vi "AO_master_CorrLoop_PD_2D_v4.vi"() -> ()   [LabVIEW 2018]
uses:
  <userlib>/WaveKit.lib/Controls/Wavefront Corrector states - ONE.ctl
  <userlib>/WaveKit.lib/Classes/WavefrontCorrector/WavefrontCorrector.lvclass
  <userlib>/WaveKit.lib/Classes/WavefrontCorrectorSet/WavefrontCorrectorSet.lvclass
  <vilib>/Analysis/1siggen.llb/Ramp Pattern by Samples.vi
  <vilib>/Utility/file.llb/Read From Spreadsheet File (DBL).vi
  <vilib>/Analysis/1siggen.llb/Ramp Pattern by Delta.vi
  <vilib>/Analysis/NI_AALBase.lvlib
panel:
  in  "Status":enum32{"Page 1", "Page 2"}(tab)
  out "DM Initial State":T1[](array[typedef])
  out "Return from CheckTimings":u32
  out "Calculated Exposure Value":sgl format="%.2f"
  out "Return from SetTemperature":u32
  out "Return from Initialize":u32
  out "Detector X Pixels":i32
  out "Detector Y Pixels":i32
  in  "Tab Control":T2(tab)
  in  "Flip mirror port":tag="Dev1/ao5"
  in  "interaction matrix file":path=path "D:/SystemAlignment/IM_20220706_1p5sx2_0p5um.aomi"
  in  "Haso configuration file":path=path "C:/Program Files (x86)/Imagine Optic/Configuration Files/HASO3_first_7364.dat"
  in  "Offset command file":path=path "D:/SystemAlignment/system_aberration_20220720.dat"
  in  "Initial haso file":path=path "D:/SystemAlignment/system_aberration_residual_20220406.has"
  out "# of Phase":i32
  in  "DM configuration file":path=path "C:/Program Files (x86)/Imagine Optic/Configuration Files/WaveFrontCorrector_mirao52-e_0326.dat"
  out "DM ActuatorsNumber":i32
  out "Error out":errorcluster
  in  "EMCCD trigger port":tag="Dev1/port0/line0"
  in  "488 shutter":refnum<k7>(container)
  in  "?":bool
  out "Flip Mirror Status":sgl(ring) items=["EMCCD Camera"=-5, "Wavefront sensor"=1]
  in  "Defocus":bool=TRUE
  in  "Tilts":bool=TRUE
  in  "Max zern num":u32=14
  in  "Density":sgl=0.3 min=0 max=1 format="%#.4f"
  in  "Amplitude":sgl=0.3 min=0 format="%#.4f"
  in  "idxType":enum16{"Wyant", "ANSI"}(ring)=enum."ANSI"
  in  "Zern coeffs file":path=path "D:/SystemAlignment/system_aberration_residual_20200711.txt"
  in  "Diversity Zern Coeffs":enum16{"Manual ", "ZernFile"}(ring)
  out "Zern coeffs (random)":sgl[](array[numeric])
  out "Zern index (random)":i32[](array[numeric])
  in  "Initial Zern Coeffs":enum16{"Manual ", "Random"}(ring)
  in  "Exp Repeat Num":i32=1
  in  "Index 5":i32[](array[numeric])=[3, 4, 5, 6, 7, 8]
  in  "Coeffs 4":sgl[](array[numeric])=[0.5, -0.2, 0.0, 0.0, 0.0, 0.0]
  in  "Index 4":i32[](array[numeric])=[3, 4, 5, 6, 7, 8]
  in  "Coeffs 3":sgl[](array[numeric])=[0.0, -0.2, 0.5, 0.0, 0.0, 0.0]
  in  "Index 3":i32[](array[numeric])=[3, 4, 5, 6, 7, 8]
  in  "Coeffs 2":sgl[](array[numeric])=[0.5, 0.2, 0.0, 0.0, 0.0, 0.0]
  in  "Index 2":i32[](array[numeric])=[3, 4, 5, 6, 7, 8]
  in  "Coeffs 5":sgl[](array[numeric])=[0.0, 0.2, 0.5, 0.0, 0.0, 0.0]
  in  "Zern index initial":i32[](array[numeric])=[3, 5, 6, 7, 12]
  in  "Zern coeffs initial":sgl[](array[numeric])=[0.0, 0.4, 0.0, 0.3, 0.0]
  out "Img Num Used":dbl[](array[numeric])
  out "Corrected IQM":dbl
  out "Recon Img Num":u32=2
  out "Current Exp Num":u32=2
  in  "Auto Stop":bool=TRUE
  in  "Feedback Type":T3(ring)=enum."One Step Feedback"
  in  "Initial Phase Num":u32=2
  out "RMSE Value":dbl
  out "Recon Time (s)":dbl
  in  "File Base Name":string="beads"
  in  "Images/phase":i32=1
  in  "Exposure time (s)":dbl=0.02
  in  "Div Phase Num":i32=5
  in  "Metrics Type":T4(ring)=enum."norm DCT  - spectral domain 3: 0~r0"
  in  "Apply Defocus":bool
  in  "PD Correction":bool=TRUE
  in  "Num for average":u32=1
  in  "Zernike Index Limit":u32=20
  in  "Max Iteration Num":u32=10
  in  "Gamma Value":dbl=1e-10
  in  "Crop Size of image":u32=512
  in  "Background Value":dbl=300.0
  in  "Show Input":bool
  in  "Show Recon":bool=TRUE
  in  "Use GPU":bool=TRUE
  out "Cooling":i32
  in  "Trigger":u32(ring)=1 items=["Internal", "External"]
  in  "Cooler set to Temperature":i32=-60
  in  "Initialize EMCCD?":bool=TRUE
  in  "Turn off EMCCD when finished?":bool
  in  "Main Path":path=path "D:/Data"
  in  "Subfolder":string="Test1"
  in  "Folder Name":string="Test"
  out "Groundtruth IQM":dbl
  out "Aberrated IQM":dbl
  out "All IQM":dbl[](array[numeric])
  in  "Final Phase Num":u32=3
  out "Output path":path=path "D:/Data"
  out "Log File Path":path
  out "Zern coeffs recon":sgl[](array[numeric])
  # "AO correction loop based on phase diversity: 2D image case (last update: 20200821)\nVersion 3: A combination of LabVIEW, MATLAB (EMCCD controlled by LabVIEW) for sensorless AO with IQM feedback , modified from Version 3. New updates:\n1) fix last 2 bugs, re-organize user interface, reform program design (framework reshaped)\n2) more control to laser and EMCCD (ROI, gain, preview)"
  # "How to use\n1) Set Flip mirror to EMCCD (AO_mini_stage and shutter control.vi);\n2) Run this VI;\n3) When cooling gets to -55, the system start to acquire data."
  # "Bugs: \n1) when run this vi first time, there is big shift between diversity images. If repeat, then shift disappears.\n2) diversity image number is not controllable, always output 5 images."
  # "Andor Status"
  # "Manual input"
  # "Random input"
  # "Manual input sequence"
  # "File input"
  # "Path and File Name"
  # "Andor EMCCD Settings"
  # "AO Correction Settings"
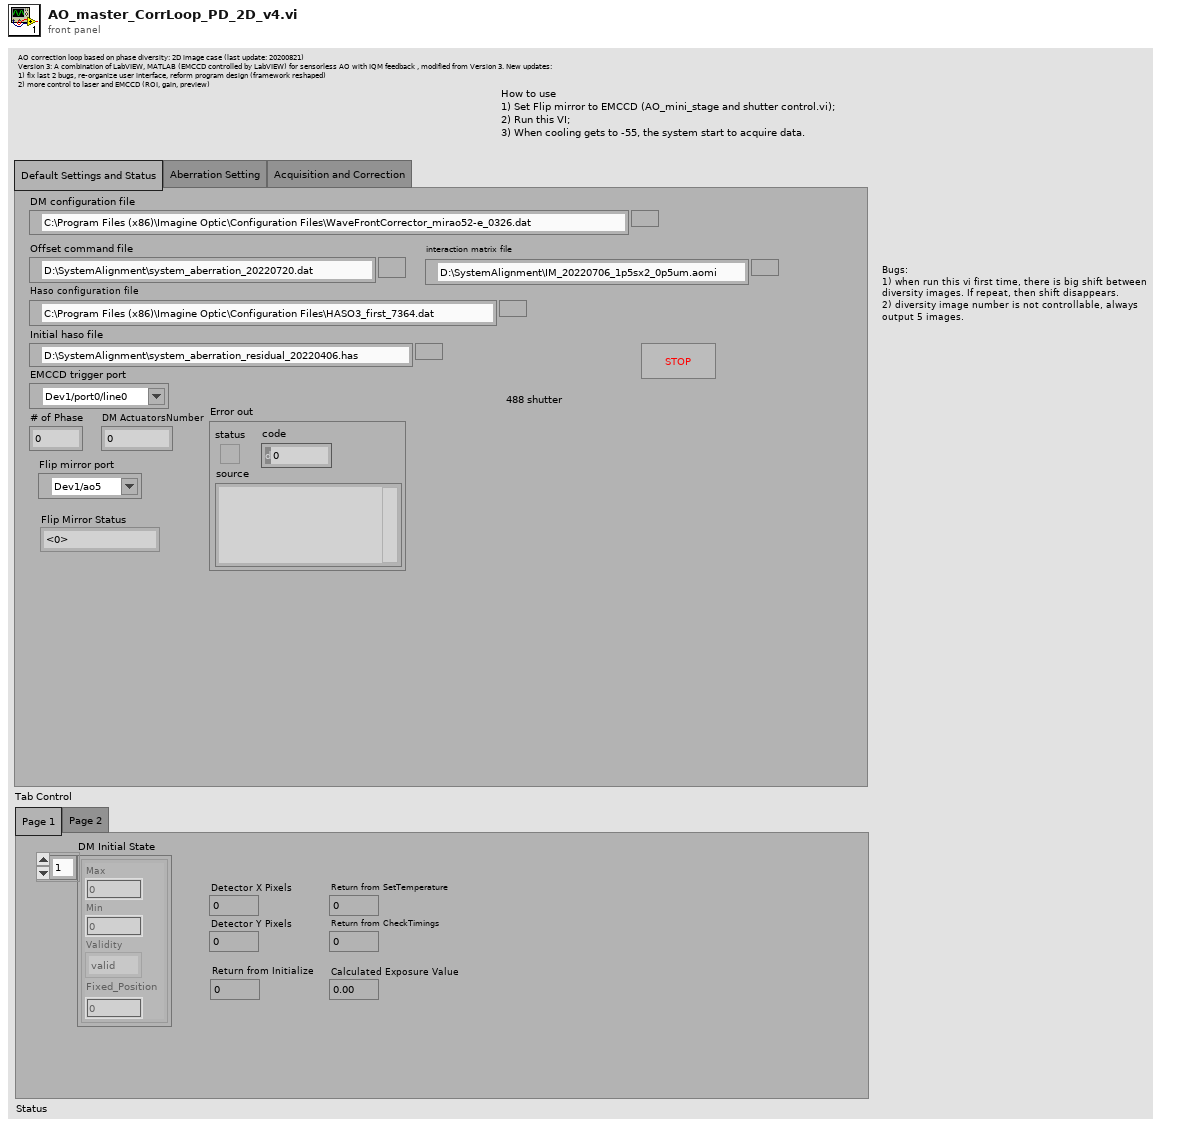
[diagram p1: front panel]
types:
  T1 = typedef "Wavefront Corrector states - ONE.ctl" = cluster{"Max":sgl, "Min":sgl, "Validity":enum16{"valid", "fixed", "invalid"}, "Fixed_Position":sgl}
  T2 = enum32{"Default Settings and Status", "Aberration Setting", "Acquisition and Correction"}
  T3 = enum16{"Single Correction", "One Step Feedback", "Progressive Feedback"}
  T4 = enum16{" ", "max intensity", "mean intensity", "RMS contrast", "sharpness - image domain", "sharpness - spectral domain 1: 0~r0", "sharpness - spectral domain 2: 0.1*r0~0.5*r0", "norm DCT  - spectral domain 3: 0~r0"}
  T5 = typedef "Error Code Enum typedef.ctl" = enum32{"N/A (0)", "DRV_ERROR_CODES", "DRV_SUCCESS", "DRV_VXDNOTINSTALLED", "DRV_ERROR_SCAN", "DRV_ERROR_CHECK_SUM", "DRV_ERROR_FILELOAD", "DRV_UNKNOWN_FUNC", "DRV_ERROR_VXD_INIT", "DRV_ERROR_ADDRESS", "DRV_ERROR_PAGELOCK", "DRV_ERROR_PAGEUNLOCK", "DRV_ERROR_BOARDTEST", "DRV_ERROR_ACK", "DRV_ERROR_UP_FIFO", "DRV_ERROR_PATTERN", "N/A (16)", "DRV_ACQUISITION_ERRORS", "DRV_ACQ_BUFFER", "DRV_ACQ_DOWNFIFO_FULL", "DRV_PROC_UNKONWN_INSTRUCTION", "DRV_ILLEGAL_OP_CODE", "DRV_KINETIC_TIME_NOT_MET", "DRV_ACCUM_TIME_NOT_MET", "DRV_NO_NEW_DATA", "N/A (25)", "DRV_SPOOLERROR", "N/A (27)", "N/A (28)", "N/A (29)", "N/A (30)", "N/A (31)", "N/A (32)", "DRV_TEMPERATURE_CODES", "DRV_TEMPERATURE_OFF", "DRV_TEMPERATURE_NOT_STABILIZED", "DRV_TEMPERATURE_STABILIZED", "DRV_TEMPERATURE_NOT_REACHED", "DRV_TEMPERATURE_OUT_RANGE", "DRV_TEMPERATURE_NOT_SUPPORTED", "DRV_TEMPERATURE_DRIFT", "N/A (41)", "N/A (42)", "N/A (43)", "N/A (44)", "N/A (45)", "N/A (46)", "N/A (47)", "N/A (48)", "DRV_GENERAL_ERRORS", "DRV_INVALID_AUX", "DRV_COF_NOTLOADED", "DRV_FPGAPROG", "DRV_FLEXERROR", "DRV_GPIBERROR", "N/A (55)", "N/A (56)", "N/A (57)", "N/A (58)", "N/A (59)", "N/A (60)", "N/A (61)", "N/A (62)", "N/A (63)", "DRV_DATATYPE", "DRV_DRIVER_ERRORS", "DRV_P1INVALID", "DRV_P2INVALID", "DRV_P3INVALID", "DRV_P4INVALID", "DRV_INIERROR", "DRV_COFERROR", "DRV_ACQUIRING", "DRV_IDLE", "DRV_TEMPCYCLE", "DRV_NOT_INITIALIZED", "DRV_P5INVALID", "DRV_P6INVALID", "DRV_INVALID_MODE", "DRV_INVALID_FILTER", "DRV_I2CERRORS", "DRV_I2CDEVNOTFOUND", "DRV_I2CTIMEOUT", "DRV_P7INVALID", "N/A (84)", "N/A (85)", "N/A (86)", "N/A (87)", "N/A (88)", "N/A (89)", "DRV_IOCERROR", "DRV_VRMVERSIONERROR"}
  T6 = typedef "NI_Matrix.lvlib/RealMatrix.ctl" = dbl[][]
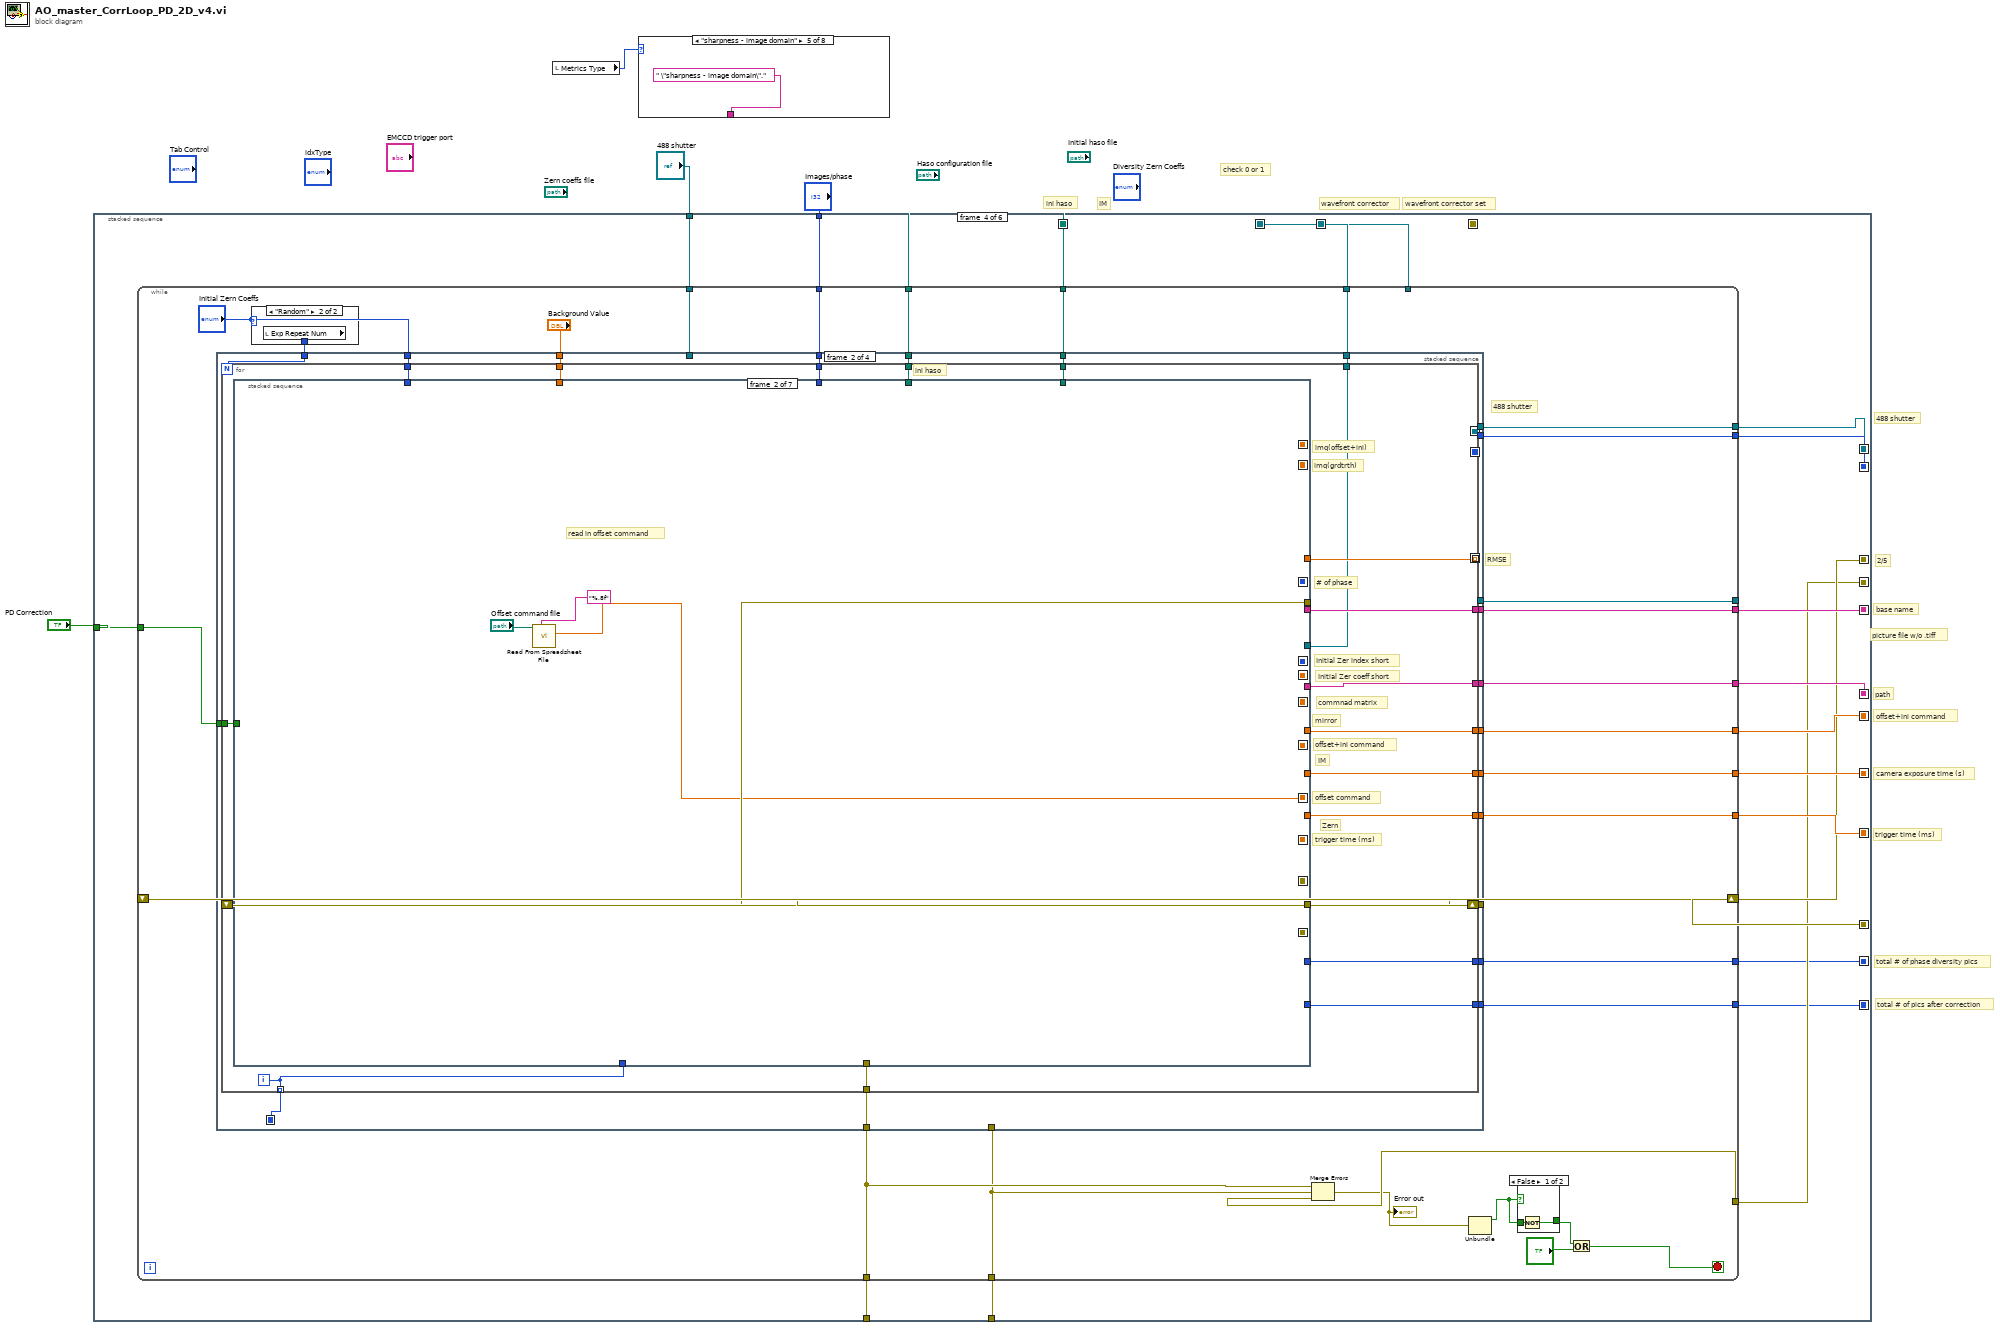
[diagram p0: block diagram]
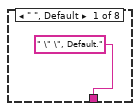
[diagram p2: hidden frame]
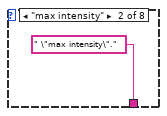
[diagram p3: hidden frame]
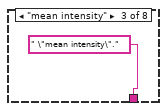
[diagram p4: hidden frame]
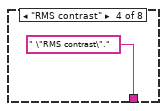
[diagram p5: hidden frame]
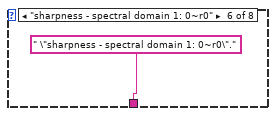
[diagram p6: hidden frame]
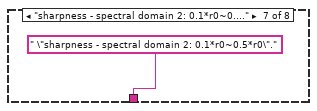
[diagram p7: hidden frame]
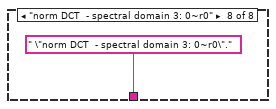
[diagram p8: hidden frame]
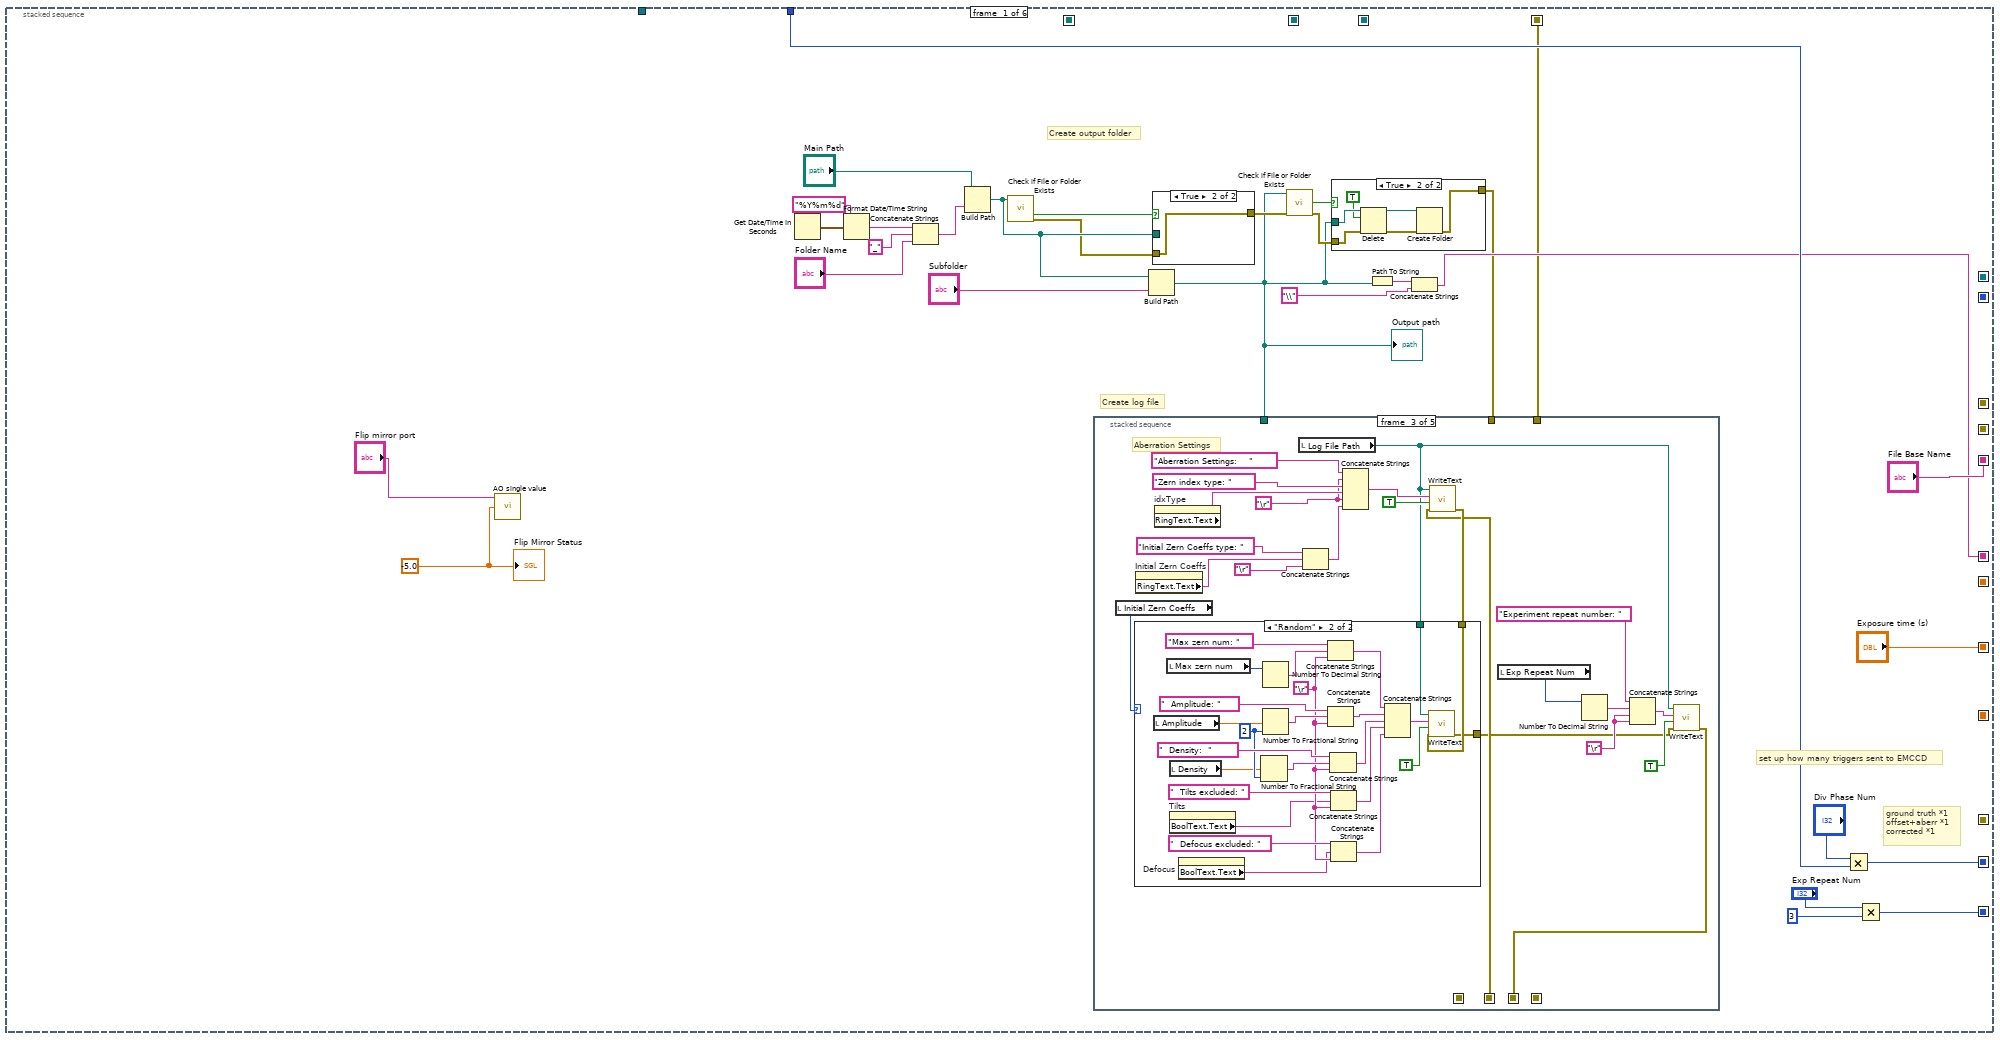
[diagram p9: hidden frame]
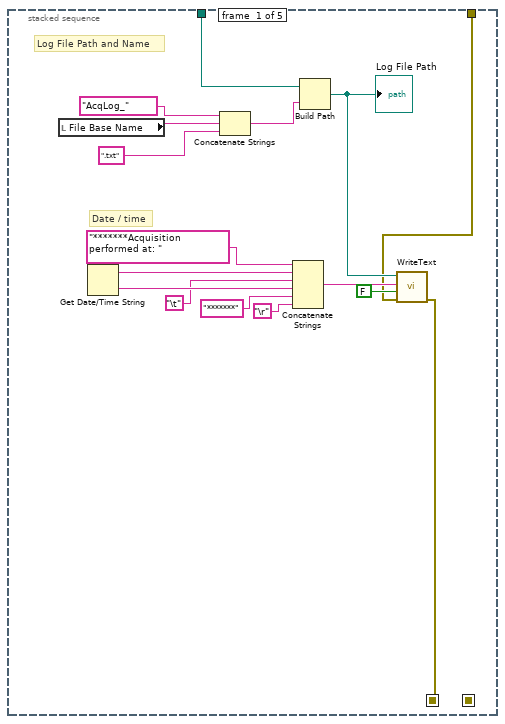
[diagram p10: hidden frame]
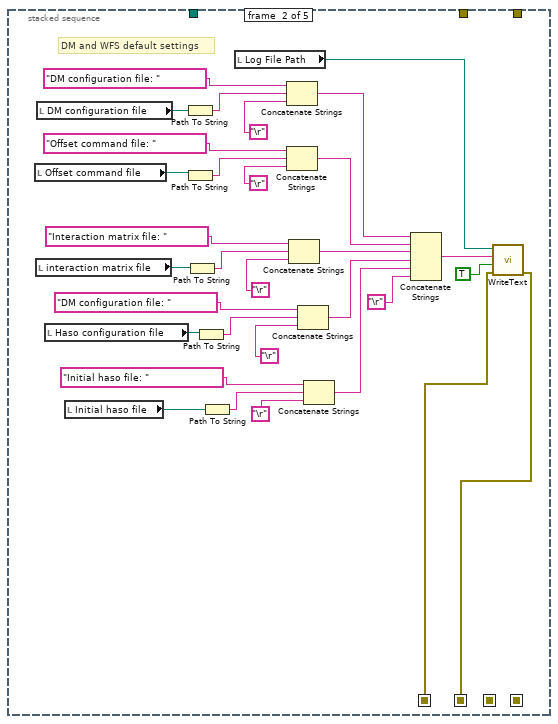
[diagram p11: hidden frame]
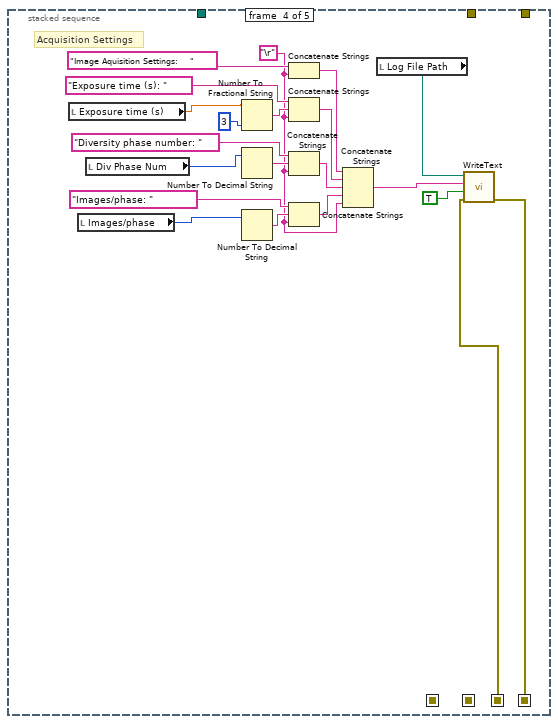
[diagram p13: hidden frame]
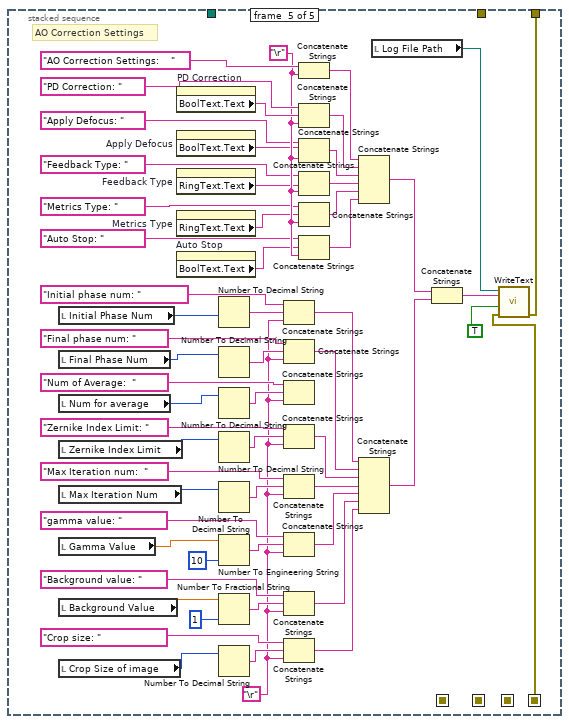
[diagram p14: hidden frame]
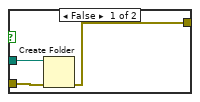
[diagram p15: hidden frame]
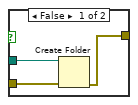
[diagram p16: hidden frame]
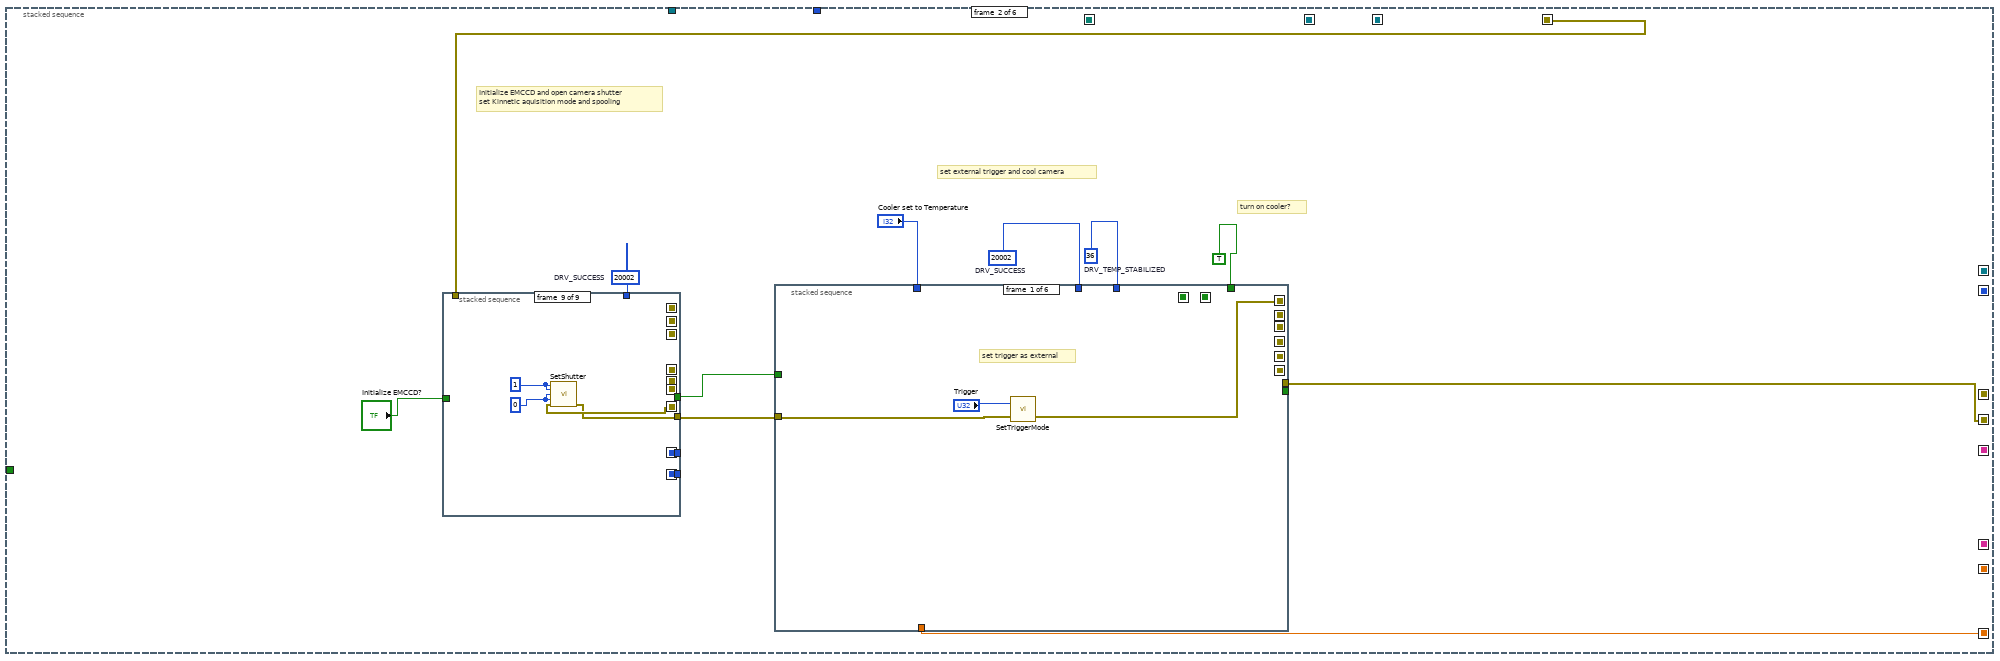
[diagram p17: hidden frame]
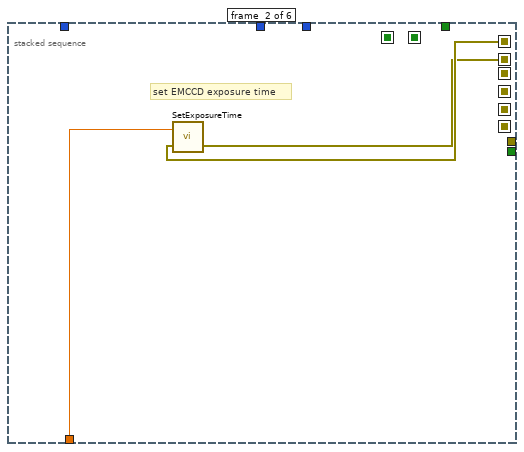
[diagram p18: hidden frame]
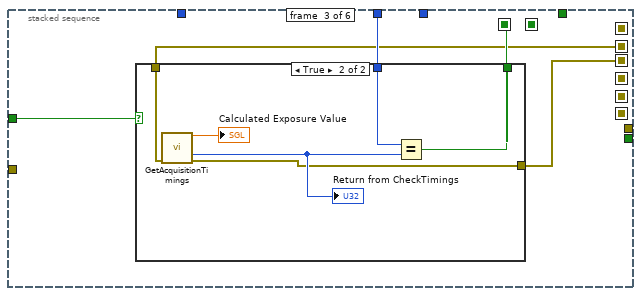
[diagram p19: hidden frame]
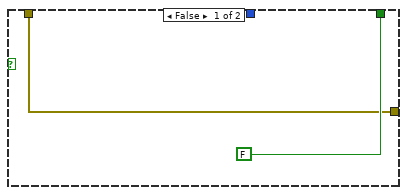
[diagram p20: hidden frame]
diagram:
  # "2/5"
  # "total # of phase diversity pics"
  # "picture file w/o .tiff"
  # "total # of pics after correction"
  # "wavefront corrector set"
  # "wavefront corrector"
  # "488 shutter"
  # "trigger time (ms)"
  # "offset+ini command"
  # "camera exposure time (s)"
  # "IM"
  # "ini haso"
  # "path"
  # "base name"
  # "check 0 or 1"
  n1 = stacked-sequence {
    seq-local: [w14 _ _ _ _ _] -> [_ _ _ w364 _ _]
    seq-local: ["File Base Name" _ _ _ _ _] -> [_ _ _ w363 _ _]
    seq-local: [_ _ w345 _ _ _] -> [_ _ _ w346 _ _]
    seq-local: ["Exposure time (s)" _ _ _ _ _] -> [_ w226 _ w362 _ _]
    seq-local: [_ _ w331 _ _ _] -> [_ _ _ w351 _ _]
    seq-local: [_ _ _ w361 _ _] -> [_ _ _ _ _ _]
    seq-local: [_ _ _ w360 _ _] -> [_ _ _ _ _ _]
    seq-local: [_ _ _ w359 _ _] -> [_ _ _ _ _ w916]
    seq-local: [_ _ _ w354 _ _] -> [_ _ _ _ _ _]
    seq-local: [_ _ _ w357 _ _] -> [_ _ _ _ _ _]
    seq-local: [_ _ w330 _ _ _] -> [_ _ _ w352 _ w918]
    seq-local: [_ _ w329 _ _ _] -> [_ _ _ w350 _ w917]
    seq-local: [w31 _ _ _ _ _] -> [_ _ _ w347 _ _]
    seq-local: [_ w227 _ _ _ _] -> [_ _ w328 w349 _ _]
    seq-local: [w30 _ _ _ _ _] -> [_ _ _ w348 _ _]
    seq-local: [w6 _ _ _ _ _] -> [_ w223 _ _ _ _]
    tunnel: "Images/phase" -> [w29 _ _ w365 _ _]
    tunnel: "PD Correction" -> [_ _ _ w358 _ _]
    tunnel: [_ _ _ w356 _ _] -> _
    tunnel: [_ _ _ w355 _ _] -> _
    tunnel: "488 shutter" -> [_ _ _ w353 _ w919]
    frame #0 {
      w12 = -5.0
      # "Create log file"
      # "Create output folder"
      # "set up how many triggers sent to EMCCD"
      # "ground truth *1\noffset+aberr *1\ncorrected *1"
      n2 = call "AO single value.vi"("data"=w12, "physical channels"="Flip mirror port") -> ()  [unwired: 1 in, 1 out]
      n3 = Get Date/Time In Seconds() -> (seconds since 1Jan1904=w24:timestamp)
      n4 = Format Date/Time String(time format string (%c)="%Y%m%d", seconds (now)=w24) -> (date/time string=w25:string)  [unwired: 1 in]
      n5 = Concatenate Strings(w25, "_", "Folder Name") -> (w26:string)
      n6 = Build Path(base path="Main Path", name or relative path=w26) -> (appended path=w28:path)
      n7 = call <vilib>:"Check if File or Folder Exists.vi"("path"=w28) -> ("error out"=w11:errorcluster, "file or folder exists?"=w22:bool)  [unwired: 8 in, 1 out]
      n8 = Build Path(base path=w28, name or relative path="Subfolder") -> (appended path=w5:path)
      "Output path" <- w5
      n9 = case shown="True" w22 {
        tunnel: w28 -> [w221 _]
        tunnel: w11 -> [w220 w222]
        tunnel: [w219 w222] -> w10
        frame False {
          n10 = Create Folder(path (use dialog)=w221, error in=w220) -> (error out=w219:errorcluster)  [unwired: 1 in, 2 out]
        }
        frame True {
        }
      }
      n11 = call <vilib>:"Check if File or Folder Exists.vi"("error in (no error)"=w10, "path"=w5) -> ("error out"=w27:errorcluster, "file or folder exists?"=w23:bool)  [unwired: 7 in, 1 out]
      n12 = case shown="True" w23 {
        tunnel: w5 -> [w212 w217]
        tunnel: w27 -> [w211 w218]
        tunnel: [w210 w213] -> w7
        frame False {
          n13 = Create Folder(path (use dialog)=w212, error in=w211) -> (error out=w210:errorcluster)  [unwired: 1 in, 2 out]
        }
        frame True {
          n14 = Delete(path (use dialog)=w217, entire hierarchy (F)=TRUE, error in=w218) -> (deleted path=w215:path, error out=w214:errorcluster)  [unwired: 2 in, 1 out]
          n15 = Create Folder(path (use dialog)=w215, error in=w214) -> (error out=w213:errorcluster)  [unwired: 1 in, 2 out]
        }
      }
      n16 = stacked-sequence {
        seq-local: [w36 _ _ _ _] -> [_ w52 _ _ _]
        seq-local: [_ w51 _ _ _] -> [_ _ w98 _ _]
        seq-local: [_ _ w85 _ _] -> [_ _ _ w133 _]
        seq-local: [_ _ _ w132 _] -> [_ _ _ _ w151]
        tunnel: w7 -> [w37 _ _ _ _]
        tunnel: [_ _ _ _ w195] -> w6
        tunnel: w5 -> [w35 _ _ _ _]
        frame #0 {
          # "Date / time"
          # "Log File Path and Name"
          n17 = local read "File Base Name"() -> (w48:string)
          n18 = Get Date/Time String() -> (date string=w45:string, time string=w44:string)  [unwired: 3 in]
          n19 = Concatenate Strings("AcqLog_", w48, ".txt") -> (w50:string)
          n20 = Concatenate Strings("*******Acquisition performed at: ", w45, "\t", w44, "*******", "\r") -> (w40:string)
          n21 = Build Path(base path=w35, name or relative path=w50) -> (appended path=w38:path)
          "Log File Path" <- w38
          n22 = call "WriteText.vi"("error in (no error)"=w37, "Appending"=FALSE, "Input Text"=w40, "File Path"=w38) -> ("error out"=w36:errorcluster)  [unwired: 7 in]
        }
        frame #1 {
          # "DM and WFS default settings"
          n23 = local read "Offset command file"() -> (w74:path)
          n24 = local read "interaction matrix file"() -> (w63:path)
          n25 = local read "DM configuration file"() -> (w79:path)
          n26 = local read "Haso configuration file"() -> (w62:path)
          n27 = local read "Initial haso file"() -> (w61:path)
          n28 = Path To String(path=w79) -> (string=w78:string)
          n29 = Path To String(path=w74) -> (string=w75:string)
          n30 = Path To String(path=w63) -> (string=w70:string)
          n31 = Path To String(path=w62) -> (string=w67:string)
          n32 = Path To String(path=w61) -> (string=w64:string)
          n33 = local read "Log File Path"() -> (w60:path)
          n34 = Concatenate Strings("DM configuration file: ", w78, "\r") -> (w58:string)
          n35 = Concatenate Strings("Offset command file: ", w75, "\r") -> (w57:string)
          n36 = Concatenate Strings("Interaction matrix file: ", w70, "\r") -> (w59:string)
          n37 = Concatenate Strings("DM configuration file: ", w67, "\r") -> (w55:string)
          n38 = Concatenate Strings("Initial haso file: ", w64, "\r") -> (w56:string)
          n39 = Concatenate Strings(w58, w57, w59, w55, w56, "\r") -> (w53:string)
          n40 = call "WriteText.vi"("error in (no error)"=w52, "Appending"=TRUE, "Input Text"=w53, "File Path"=w60) -> ("error out"=w51:errorcluster)  [unwired: 7 in]
        }
        frame #2 {
          w87 = "\r"
          w82 = "\r"
          # "Aberration Settings"
          n41 = local read "Initial Zern Coeffs"() -> (w93:enum16{"Manual ", "Random"})
          n42 = property on="Initial Zern Coeffs" class="Enum (strict)"() -> ("RingText.Text"=w95:string)  [unwired: 2 in, 2 out]
          n43 = property on="idxType" class="Enum (strict)"() -> ("RingText.Text"=w99:string)  [unwired: 2 in, 2 out]
          n44 = local read "Log File Path"() -> (w84:path)
          n45 = Concatenate Strings("Initial Zern Coeffs type: ", w95, "\r") -> (w94:string)
          n46 = Concatenate Strings("Aberration Settings:    ", w82, "Zern index type: ", w99, w82, w94) -> (w101:string)
          n47 = call "WriteText.vi"("error in (no error)"=w98, "Appending"=TRUE, "Input Text"=w101, "File Path"=w84) -> ("error out"=w100:errorcluster)  [unwired: 7 in]
          n48 = case shown="\"Random\"" w93 {
            tunnel: w84 -> [_ w125]
            tunnel: w100 -> [w104 w124]
            tunnel: [w104 w123] -> w86
            frame "Manual ", Default {
            }
            frame "Random" {
              w116 = 2
              w109 = "\r"
              n49 = local read "Amplitude"() -> (w127:sgl)
              n50 = local read "Max zern num"() -> (w126:u32)
              n51 = local read "Density"() -> (w115:sgl)
              n52 = property on="Tilts" class="Bool (strict)"() -> ("BoolText.Text"=w108:string)  [unwired: 2 in, 2 out]
              n53 = property on="Defocus" class="Bool (strict)"() -> ("BoolText.Text"=w107:string)  [unwired: 2 in, 2 out]
              n54 = Number To Fractional String(number=w115, precision (6)=w116) -> (F-format string=w117:string)  [unwired: 2 in]
              n55 = Number To Decimal String(number=w126) -> (decimal integer string=w121:string)  [unwired: 1 in]
              n56 = Number To Fractional String(number=w127, precision (6)=w116) -> (F-format string=w119:string)  [unwired: 2 in]
              n57 = Concatenate Strings("Max zern num: ", w121, w109) -> (w114:string)
              n58 = Concatenate Strings("  Amplitude: ", w119, w109) -> (w113:string)
              n59 = Concatenate Strings("  Density:  ", w117, w109) -> (w112:string)
              n60 = Concatenate Strings("  Tilts excluded: ", w108, w109) -> (w105:string)
              n61 = Concatenate Strings("  Defocus excluded: ", w107, w109) -> (w106:string)
              n62 = Concatenate Strings(w114, w113, w112, w105, w106) -> (w128:string)
              n63 = call "WriteText.vi"("error in (no error)"=w124, "Appending"=TRUE, "Input Text"=w128, "File Path"=w125) -> ("error out"=w123:errorcluster)  [unwired: 7 in]
            }
          }
          n64 = local read "Exp Repeat Num"() -> (w89:i32)
          n65 = Number To Decimal String(number=w89) -> (decimal integer string=w90:string)  [unwired: 1 in]
          n66 = Concatenate Strings("Experiment repeat number: ", w90, w87, w87) -> (w91:string)
          n67 = call "WriteText.vi"("error in (no error)"=w86, "Appending"=TRUE, "Input Text"=w91, "File Path"=w84) -> ("error out"=w85:errorcluster)  [unwired: 7 in]
        }
        frame #3 {
          w130 = "\r"
          # "Acquisition Settings"
          n68 = local read "Exposure time (s)"() -> (w135:dbl)
          n69 = local read "Images/phase"() -> (w137:i32)
          n70 = local read "Div Phase Num"() -> (w139:i32)
          n71 = Number To Fractional String(number=w135, precision (6)=3) -> (F-format string=w131:string)  [unwired: 2 in]
          n72 = Number To Decimal String(number=w139) -> (decimal integer string=w148:string)  [unwired: 1 in]
          n73 = Number To Decimal String(number=w137) -> (decimal integer string=w147:string)  [unwired: 1 in]
          n74 = Concatenate Strings("Image Aquisition Settings:    ", w130) -> (w146:string)
          n75 = Concatenate Strings("Exposure time (s): ", w131, w130) -> (w145:string)
          n76 = Concatenate Strings("Diversity phase number: ", w148, w130) -> (w144:string)
          n77 = Concatenate Strings("Images/phase: ", w147, w130) -> (w143:string)
          n78 = Concatenate Strings(w146, w145, w144, w143, w130) -> (w136:string)
          n79 = local read "Log File Path"() -> (w149:path)
          n80 = call "WriteText.vi"("error in (no error)"=w133, "Appending"=TRUE, "Input Text"=w136, "File Path"=w149) -> ("error out"=w132:errorcluster)  [unwired: 7 in]
        }
        frame #4 {
          w162 = "\r"
          w192 = "\r"
          # "AO Correction Settings"
          n81 = local read "Initial Phase Num"() -> (w201:u32)
          n82 = local read "Final Phase Num"() -> (w199:u32)
          n83 = local read "Num for average"() -> (w176:u32)
          n84 = local read "Zernike Index Limit"() -> (w173:u32)
          n85 = local read "Max Iteration Num"() -> (w170:u32)
          n86 = local read "Gamma Value"() -> (w198:dbl)
          n87 = local read "Background Value"() -> (w166:dbl)
          n88 = local read "Crop Size of image"() -> (w163:u32)
          n89 = property on="PD Correction" class="Bool (strict)"() -> ("BoolText.Text"=w194:string)  [unwired: 2 in, 2 out]
          n90 = property on="Apply Defocus" class="Bool (strict)"() -> ("BoolText.Text"=w191:string)  [unwired: 2 in, 2 out]
          n91 = property on="Feedback Type" class="Enum (strict)"() -> ("RingText.Text"=w189:string)  [unwired: 2 in, 2 out]
          n92 = property on="Metrics Type" class="Enum (strict)"() -> ("RingText.Text"=w187:string)  [unwired: 2 in, 2 out]
          n93 = property on="Auto Stop" class="Bool (strict)"() -> ("BoolText.Text"=w185:string)  [unwired: 2 in, 2 out]
          n94 = Number To Decimal String(number=w201) -> (decimal integer string=w207:string)  [unwired: 1 in]
          n95 = Number To Decimal String(number=w199) -> (decimal integer string=w206:string)  [unwired: 1 in]
          n96 = Number To Decimal String(number=w176) -> (decimal integer string=w178:string)  [unwired: 1 in]
          n97 = Number To Decimal String(number=w173) -> (decimal integer string=w175:string)  [unwired: 1 in]
          n98 = Number To Decimal String(number=w170) -> (decimal integer string=w172:string)  [unwired: 1 in]
          n99 = Number To Engineering String(2:10, 4:w198) -> (0:w196:string)  [unwired: 2 in]
          n100 = Number To Fractional String(number=w166, precision (6)=1) -> (F-format string=w167:string)  [unwired: 2 in]
          n101 = Number To Decimal String(number=w163) -> (decimal integer string=w165:string)  [unwired: 1 in]
          n102 = Concatenate Strings("Initial phase num: ", w207, w162) -> (w161:string)
          n103 = Concatenate Strings("Final phase num: ", w206, w162) -> (w160:string)
          n104 = Concatenate Strings("Num of Average:  ", w178, w162) -> ()  [unwired: 1 out]
          n105 = Concatenate Strings("Zernike Index Limit: ", w175, w162) -> (w159:string)
          n106 = Concatenate Strings("Max Iteration num:  ", w172, w162) -> (w155:string)
          n107 = Concatenate Strings("gamma value: ", w196, w162) -> (w156:string)
          n108 = Concatenate Strings("Background value: ", w167, w162) -> (w157:string)
          n109 = Concatenate Strings("Crop size: ", w165, w162) -> (w158:string)
          n110 = Concatenate Strings("AO Correction Settings:    ", w192) -> (w205:string)
          n111 = Concatenate Strings("PD Correction: ", w194, w192) -> (w183:string)
          n112 = Concatenate Strings("Apply Defocus: ", w191, w192) -> (w182:string)
          n113 = Concatenate Strings("Feedback Type: ", w189, w192) -> (w179:string)
          n114 = Concatenate Strings("Metrics Type: ", w187, w192) -> (w180:string)
          n115 = Concatenate Strings("Auto Stop: ", w185, w192) -> (w181:string)
          n116 = Concatenate Strings(w205, w183, w182, w179, w180, w181) -> (w153:string)
          n117 = Concatenate Strings(w161, w160, w159, w155, w156, w157, w158) -> (w152:string)
          n118 = local read "Log File Path"() -> (w208:path)
          n119 = Concatenate Strings(w153, w152) -> (w154:string)
          n120 = call "WriteText.vi"("error in (no error)"=w151, "Appending"=TRUE, "Input Text"=w154, "File Path"=w208) -> ("error out"=w195:errorcluster)  [unwired: 7 in]
        }
      }
      n121 = Path To String(path=w5) -> (string=w16:string)
      n122 = Concatenate Strings(w16, "\\") -> (w14:string)
      n123 = Multiply(x="Div Phase Num", y=w29) -> (x*y=w30:i32)
      n124 = Multiply(x="Exp Repeat Num", y=3) -> (x*y=w31:i32)
      "Flip Mirror Status" <- w12
    }
    frame #1 {
      w229 = 36  # DRV_TEMP_STABILIZED
      w231 = 20002  # DRV_SUCCESS
      w233 = 20002  # DRV_SUCCESS
      # "turn on cooler?"
      # "set external trigger and cool camera"
      # "Initialize EMCCD and open camera shutter\nset Kinnetic aquisition mode and spooling"
      n125 = stacked-sequence {
        seq-local: [_ _ _ _ _ _ _ w317 _] -> [_ _ _ _ _ _ _ _ _]
        seq-local: [_ _ _ _ _ _ _ w319 _] -> [_ _ _ _ _ _ _ _ _]
        seq-local: [w287 _ _ _ _ _ _ _ _] -> [_ _ w300 _ _ _ _ _ _]
        seq-local: [_ _ w299 _ _ _ _ _ _] -> [_ _ _ w303 _ _ _ _ _]
        seq-local: [_ _ _ w302 _ _ _ _ _] -> [_ _ _ _ w305 _ _ _ _]
        seq-local: [_ _ _ _ w306 _ _ _ _] -> [_ _ _ _ _ w309 _ _ _]
        seq-local: [_ _ _ _ _ w308 _ _ _] -> [_ _ _ _ _ _ w313 _ _]
        seq-local: [_ _ _ _ _ _ w311 _ _] -> [_ _ _ _ _ _ _ w322 _]
        seq-local: [_ _ _ _ _ _ _ w320 _] -> [_ _ _ _ _ _ _ _ w325]
        tunnel: w233 -> [w289 _ _ _ _ _ _ _ _]
        tunnel: [w288 _ _ _ _ _ _ _ _] -> w232
        tunnel: [_ _ _ _ _ _ _ w317 _] -> _
        tunnel: [_ _ _ _ _ _ _ w319 _] -> _
        tunnel: [_ _ _ _ _ _ _ _ w324] -> w228
        tunnel: "Initialize EMCCD?" -> [w286 _ _ _ _ _ _ _ _]
        tunnel: w223 -> [w285 _ _ _ _ _ _ _ _]
        frame #0 {
          # "Initialize EMCCD"
          n126 = case shown="True" w286 {
            tunnel: w289 -> [_ w295]
            tunnel: [TRUE w294] -> w288
            tunnel: [errorcluster {"status"=FALSE, "code"=0, "source"=""} ("Error in 2") w293] -> w287
            tunnel: w285 -> [_ w292]
            frame False {
            }
            frame True {
              n127 = call <userlib>:"Initialize.vi"("error in (no error)"=w292, "directory (\"\")"="" ("directory (\"\")")) -> ("error out"=w293:errorcluster, "DLL error code"=w297:u32)
              "Return from Initialize" <- w297
              n128 = Equal?(x=w295, y=w297) -> (x = y?=w294:bool)
            }
          }
        }
        frame #1 {
          # "It's 2 seconds in andor example vi"
          n129 = Wait (ms)(milliseconds to wait=u32 500) -> ()  [unwired: 1 out]
        }
        frame #2 {
          w301 = u16 4  # ReadMode: Image
          n130 = call <userlib>:"SetReadMode.vi"("error in (no error)"=w300, "mode"=w301) -> ("error out"=w299:errorcluster)  [unwired: 1 out]
        }
        frame #3 {
          w304 = u16 3  # AcquisitionMode: Kinetics
          n131 = call <userlib>:"SetAcquisitionMode.vi"("error in (no error)"=w303, "mode"=w304) -> ("error out"=w302:errorcluster)  [unwired: 1 out]
        }
        frame #4 {
          n132 = call <userlib>:"SetADChannel.vi"("error in (no error)"=w305, "channel"=0) -> ("error out"=w306:errorcluster)  [unwired: 1 out]
        }
        frame #5 {
          w310 = 0
          n133 = call <userlib>:"SetHSSpeed.vi"("error in (no error)"=w309, "index"=w310, "type"=w310) -> ("error out"=w308:errorcluster)  [unwired: 1 in, 1 out]
        }
        frame #6 {
          n134 = call <userlib>:"GetNumberVSSpeeds.vi"("error in (no error)"=w313) -> ("error out"=w312:errorcluster, "number"=w316:i32)  [unwired: 2 in, 1 out]
          n135 = Subtract(x=w316, y=1) -> (x-y=w314:i32)
          n136 = call <userlib>:"SetVSSpeed.vi"("error in (no error)"=w312, "index"=w314) -> ("error out"=w311:errorcluster)  [unwired: 1 out]
        }
        frame #7 {
          w323 = 1
          n137 = call <userlib>:"GetDetector.vi"("error in (no error)"=w322) -> ("error out"=w321:errorcluster, "ypixels"=w318:i32, "xpixels"=w319:i32)  [unwired: 3 in, 1 out]
          "Detector Y Pixels" <- w318
          "Detector X Pixels" <- w319
          n138 = Max & Min(x=w319, y=w318) -> (min(x,y)=w317:i32)  [unwired: 1 out]
          n139 = call <userlib>:"SetImage.vi"("hbin"=w323, "vbin"=w323, "hstart"=w323, "hend"=w317, "vstart"=w323, "vend"=w317, "error in (no error)"=w321) -> ("error out"=w320:errorcluster)  [unwired: 19 in, 1 out]
        }
        frame #8 {
          w326 = 0
          w327 = 1
          n140 = call <userlib>:"SetShutter.vi"("type"=w327, "mode"=w327, "closingtime"=w326, "openingtime"=w326, "error in (no error)"=w325) -> ("error out"=w324:errorcluster)  [unwired: 9 in, 1 out]
        }
      }
      n141 = stacked-sequence {
        seq-local: [_ _ w242 _ _ _] -> [_ _ _ _ _ _]
        seq-local: [_ _ _ w255 _ _] -> [_ _ _ _ _ _]
        seq-local: [w234 _ _ _ _ _] -> [_ w239 _ _ _ _]
        seq-local: [_ w238 _ _ _ _] -> [_ _ w241 _ _ _]
        seq-local: [_ _ w240 _ _ _] -> [_ _ _ w254 _ _]
        seq-local: [_ _ _ w253 _ _] -> [_ _ _ _ w261 _]
        seq-local: [_ _ _ _ w260 _] -> [_ _ _ _ _ w267]
        seq-local: [_ _ _ _ _ w265] -> [_ _ _ _ _ _]
        tunnel: w231 -> [_ _ w244 w258 _ _]
        tunnel: "Cooler set to Temperature" -> [_ _ _ w256 _ w268]
        tunnel: w229 -> [_ _ _ _ _ w269]
        tunnel: [_ _ _ w255 _ _] -> _
        tunnel: w232 -> [_ _ w243 _ _ _]
        tunnel: w228 -> [w235 _ _ _ _ _]
        tunnel: [_ _ _ _ _ w265] -> w227
        tunnel: w226 -> [_ w237 _ _ _ _]
        tunnel: TRUE -> [_ _ _ _ w259 w266]
        frame #0 {
          # "set trigger as external"
          n142 = call <userlib>:"SetTriggerMode.vi"("error in (no error)"=w235, "mode"="Trigger") -> ("error out"=w234:errorcluster)  [unwired: 1 out]
        }
        frame #1 {
          # "set EMCCD exposure time"
          n143 = call <userlib>:"SetExposureTime.vi"("error in (no error)"=w239, "time"=w237) -> ("error out"=w238:errorcluster)  [unwired: 1 out]
        }
        frame #2 {
          n144 = case shown="True" w243 {
            tunnel: w244 -> [_ w250]
            tunnel: [FALSE w252] -> w242
            tunnel: w241 -> [w245 w248]
            tunnel: [w245 w247] -> w240
            frame False {
            }
            frame True {
              n145 = call <userlib>:"GetAcquisitionTimings.vi"("error in (no error)"=w248) -> ("exposure"=→"Calculated Exposure Value":sgl, "DLL error code"=w249:u32, "error out"=w247:errorcluster)  [unwired: 10 in, 2 out]
              "Return from CheckTimings" <- w249
              n146 = Equal?(x=w250, y=w249) -> (x = y?=w252:bool)
            }
          }
        }
        frame #3 {
          # "set camera temperature to -60C"
          n147 = call <userlib>:"SetTemperature.vi"("error in (no error)"=w254, "temperature"=w256) -> ("error out"=w253:errorcluster, "DLL error code"=w257:u32)
          "Return from SetTemperature" <- w257
          n148 = Equal?(x=w258, y=w257) -> (x = y?=w255:bool)
        }
        frame #4 {
          # "turn on cooler"
          n149 = case shown="True" w259 {
            tunnel: w261 -> [w262 w264]
            tunnel: [w262 w263] -> w260
            frame False {
            }
            frame True {
              n150 = call <userlib>:"CoolerON.vi"("error in (no error)"=w264) -> ("error out"=w263:errorcluster)  [unwired: 1 in, 1 out]
            }
          }
        }
        frame #5 {
          # "wait the camera to cool down,\nwill not move forward untill the temperature reach 60C"
          n151 = case shown="True" w266 {
            tunnel: w269 -> [_ w274]
            tunnel: w268 -> [_ w273]
            tunnel: w267 -> [w270 w272]
            tunnel: [w270 w271] -> w265
            frame False {
            }
            frame True {
              n152 = while {
                tunnel: w274 -> [w283]
                tunnel: w273 -> [w278]
                tunnel: w272 -> [w281]
                tunnel: [w280] -> w271
                stop <- w275 continue-if-true
                n153 = Wait Until Next ms Multiple(millisecond multiple=u32 500) -> ()  [unwired: 1 out]
                n154 = call <userlib>:"GetTemperature.vi"("error in (no error)"=w281) -> ("error out"=w280:errorcluster, "status"=w282:T5, "temperature"=w276:i32)  [unwired: 3 in, 1 out]
                "Cooling" <- w276
                n155 = Add(x=w278, y=5) -> (x+y=w277:i32)
                n156 = Not Equal?(x=w283, y=w282) -> ()  [unwired: 1 out]
                n157 = Greater?(x=w276, y=w277) -> (0:w275:bool)
              }
            }
          }
        }
      }
    }
    frame #2 {
      # "Initialize CASAO"
      n158 = call <userlib>:"LVClass_WavefrontCorrectorSet ctor.vi"("WavefrontCorrectorSet in"=refnum<class "WavefrontCorrectorSet.lvclass"> refnum, "PathToWavefrontCorrectorSetupFile"="DM configuration file", "error in (no error)"=w328) -> ("WavefrontCorrectorSet out"=w335:refnum<class "WavefrontCorrectorSet.lvclass">, "error out"=w344:errorcluster)  [unwired: 11 in]
      n159 = call <userlib>:"LVClass_WavefrontCorrector ctor.vi"("WavefrontCorrector in"=refnum<class "WavefrontCorrector.lvclass"> refnum, "PathToWavefrontCorrectorSetupFile"="DM configuration file", "error in (no error)"=w344) -> ("WavefrontCorrector out"=w339:refnum<class "WavefrontCorrector.lvclass">, "error out"=w338:errorcluster)  [unwired: 11 in]
      n160 = call <userlib>:"LVClass_WavefrontCorrector Init.vi"("WavefrontCorrector in"=w339, "set_init_state_from_config_file"=TRUE, "error in (no error)"=w338) -> ("WavefrontCorrector out"=w333:refnum<class "WavefrontCorrector.lvclass">, "error out"=w337:errorcluster)  [unwired: 11 in]
      n161 = call <userlib>:"LVClass_WavefrontCorrectorSet get nb of actuators.vi"("WavefrontCorrectorSet in"=w335, "error in (no error)"=w337) -> ("WavefrontCorrectorSet out"=w329:refnum<class "WavefrontCorrectorSet.lvclass">, "ActuatorsNumber"=→"DM ActuatorsNumber":i32, "error out"=w334:errorcluster)  [unwired: 11 in]
      n162 = call <userlib>:"LVClass_WavefrontCorrector Get Current Preferences.vi"("WavefrontCorrector in"=w333, "error in (no error)"=w334) -> ("WavefrontCorrector out"=w330:refnum<class "WavefrontCorrector.lvclass">, "Mirror preferences.Wavefront Corrector State"=→"DM Initial State":T1[], "error out"=w331:errorcluster)  [unwired: 10 in, 1 out]
      n163 = local read "Initial haso file"() -> (w345:path)
    }
    frame #3 {
      n164 = while {
        tunnel: w365 -> [w394]
        tunnel: w364 -> [w393]
        tunnel: w363 -> [w392]
        tunnel: w346 -> [w391]
        tunnel: w362 -> [w390]
        tunnel: [w388] -> w361
        tunnel: [w387] -> w360
        tunnel: w358 -> [w385]
        tunnel: [w384] -> w357
        tunnel: [w383] -> _
        tunnel: [w381] -> w356
        tunnel: [w382] -> w355
        shift-right: [w386] -> w359
        shift-left: w351 -> [w389]
        tunnel: [w380] -> w354
        tunnel: w353 -> [w379]
        tunnel: w352 -> [w378]
        tunnel: w350 -> [_]
        tunnel: w349 -> [w376]
        tunnel: w348 -> [w370]
        tunnel: w347 -> [w369]
        tunnel: w346 -> [w367]
        stop <- w372 stop-if-true
        # "488 shutter"
        # "RMSE"
        n165 = case shown="\"Random\"" "Initial Zern Coeffs" {
          tunnel: [1 w396] -> w377
          frame "Manual ", Default {
          }
          frame "Random" {
            n166 = local read "Exp Repeat Num"() -> (w396:i32)
          }
        }
        n167 = stacked-sequence {
          seq-local: [_ w416 _ _] -> [_ _ _ w908]
          seq-local: [_ w415 _ _] -> [_ _ _ _]
          seq-local: [w402 _ _ _] -> [_ _ w904 _]
          seq-local: [w403 _ _ _] -> [_ _ w903 _]
          tunnel: w394 -> [_ w427 _ _]
          tunnel: w393 -> [_ w426 _ w907]
          tunnel: w392 -> [_ w425 _ w906]
          tunnel: w391 -> [_ w424 _ _]
          tunnel: w390 -> [_ w423 _ _]
          tunnel: w389 -> [_ w422 _ _]
          tunnel: [_ w421 _ _] -> w388
          tunnel: [_ w420 _ _] -> w387
          tunnel: [_ w419 _ _] -> w386
          tunnel: w385 -> [_ w418 _ _]
          tunnel: w377 -> [_ w417 _ _]
          tunnel: [_ _ w902 _] -> w383
          tunnel: [_ _ w901 _] -> w384
          tunnel: [_ _ _ w905] -> w381
          tunnel: [_ w414 _ _] -> w382
          tunnel: [w402 _ _ _] -> w380
          tunnel: w379 -> [w401 _ _ _]
          tunnel: w378 -> [_ w413 _ _]
          tunnel: w370 -> [_ w412 _ _]
          tunnel: w369 -> [_ w411 _ _]
          tunnel: "Background Value" -> [_ w410 _ _]
          tunnel: w367 -> [_ w409 _ _]
          tunnel: "Initial Zern Coeffs" -> [_ w408 _ _]
          frame #0 {
            # "open the shutter of 488nm laser"
            n168 = property class="MG17Motor"(reference=w401, "HWSerialNum"=85819115.0) -> (reference out=w407:refnum<k7>)  [unwired: 1 in, 1 out]
            n169 = invoke class="MG17Motor" method="StartCtrl"(reference=w407) -> (reference out=w405:refnum<k7>)  [unwired: 2 in, 2 out]
            n170 = Wait (ms)(milliseconds to wait=1000) -> ()  [unwired: 1 out]
            n171 = invoke class="MG17Motor" method="SC_Enable"(reference=w405, "lChanID"=0) -> (reference out=w402:refnum<k7>, "lChanID"=w403:i32)  [unwired: 2 in, 2 out]
          }
          frame #1 {
            n172 = for {
              N: w417 -> [_]
              tunnel: w427 -> [w446]
              tunnel: w426 -> [w445]
              tunnel: w425 -> [w444]
              tunnel: w424 -> [w443]
              tunnel: w423 -> [w442]
              tunnel: [w440] -> w421
              tunnel: [w439] -> w420
              tunnel: w418 -> [w437]
              shift-right: [w438] -> w419
              shift-left: w422 -> [w441]
              tunnel: [w436] -> w416 mode=indexing
              tunnel: [w435] -> w415 mode=indexing
              tunnel: [w434] -> w414
              tunnel: w413 -> [w433]
              tunnel: w412 -> [w432]
              tunnel: w411 -> [w431]
              tunnel: w410 -> [w430]
              tunnel: w409 -> [w429]
              tunnel: w408 -> [w428]
              i -> [w435]
              # "imq(grdtrth)"
              # "imq(offset+ini)"
              # "# of phase"
              # "trigger time (ms)"
              # "offset+ini command"
              # "Initial Zer coeff short"
              # "Initial Zer index short"
              # "mirror"
              # "Zern"
              # "commnad matrix"
              # "ini haso"
              # "IM"
              # "offset command"
              n173 = stacked-sequence {
                seq-local: [_ w462 _ _ _ _ _] -> [_ _ w480 _ w616 w674 _]
                seq-local: [_ _ w478 _ _ _ _] -> [_ _ _ w603 _ w676 _]
                seq-local: [_ _ w476 _ _ _ _] -> [_ _ _ w608 _ _ _]
                seq-local: [_ _ w471 _ _ _ _] -> [_ _ _ w605 _ _ _]
                seq-local: [w451 _ _ _ _ _ _] -> [_ _ w468 _ _ _ _]
                seq-local: [w450 _ _ _ _ _ _] -> [_ _ w467 _ _ _ _]
                seq-local: [_ _ w466 _ _ _ _] -> [_ _ _ _ w618 w680 _]
                seq-local: [_ _ _ w606 _ _ _] -> [_ _ _ _ w621 w668 _]
                seq-local: [_ _ _ w604 _ _ _] -> [_ _ _ _ _ w678 _]
                seq-local: [_ _ _ _ w617 _ _] -> [_ _ _ _ _ _ _]
                seq-local: [_ _ _ _ w615 _ _] -> [_ _ _ _ _ w669 _]
                tunnel: w446 -> [_ _ w473 w607 _ w679 _]
                tunnel: w445 -> [_ _ w474 w595 w624 w681 _]
                tunnel: w444 -> [_ _ w475 w594 w623 w682 _]
                tunnel: w443 -> [_ _ _ _ _ w666 _]
                tunnel: w442 -> [_ _ _ w614 _ _ _]
                tunnel: w441 -> [_ _ w472 _ _ _ _]
                tunnel: [_ _ _ w604 _ _ _] -> w438
                tunnel: [_ _ w466 _ _ _ _] -> w440
                tunnel: [_ _ _ w606 _ _ _] -> w439
                tunnel: w437 -> [_ _ _ _ _ w677 _]
                tunnel: w435 -> [w448 _ w465 w597 w622 w667 w899]
                tunnel: [_ _ _ _ _ w675 _] -> w436
                tunnel: [_ _ _ _ _ w673 _] -> w434
                tunnel: w433 -> [_ _ _ w609 w620 w672 _]
                tunnel: w432 -> [_ _ _ _ _ _ _]
                tunnel: w431 -> [_ _ _ _ _ w671 _]
                tunnel: w430 -> [_ _ _ _ w619 w670 _]
                tunnel: w429 -> [_ _ _ _ _ w665 _]
                tunnel: w428 -> [w447 _ _ _ _ _ _]
                frame #0 {
                  # "generate initial aberration (aberr to correct)"
                  n174 = case shown="\"Manual \"" w447 {
                    tunnel: ["Zern index initial" w461] -> w451
                    tunnel: ["Zern coeffs initial" w460] -> w450
                    frame "Manual " {
                    }
                    frame "Random" {
                      # "generate random zernike index and coefficient arrays"
                      n175 = local read "idxType"() -> (w458:enum16{"Wyant", "ANSI"})
                      n176 = call "zerncoeffs_RDgenerator.vi"("Defocus"="Defocus", "Tilts"="Tilts", "idxType"=w458, "Density"="Density", "Aplitude"="Amplitude", "Max zern num"="Max zern num") -> ("Zern coeff"=w460:sgl[], "Zern index"=w461:i32[])  [unwired: 4 in]
                      "Zern index (random)" <- w461
                      "Zern coeffs (random)" <- w460
                    }
                  }
                  n177 = Increment(x=w448) -> (x+1=→"Current Exp Num":i32)
                }
                frame #1 {
                  # "read in offset command"
                  n178 = call-poly <vilib>:"Read From Spreadsheet File.vi"("format (%.3f)"="%.8f", "file path (dialog if empty)"="Offset command file") -> ("first row"=w462:dbl[])  [unwired: 5 in, 4 out]
                }
                frame #2 {
                  w485 = 0.0
                  # "ini zern coeff"
                  # "offset+ini command"
                  # "Zern coeff"
                  # "Zern index"
                  # "calculate the command:\nfor phase diversity"
                  n179 = Array Size(array="Index 2") -> (size(s)=w483:i32)
                  n180 = call-poly <vilib>:"Ramp Pattern.vi"("start"=w485, "end"=w485, "samples"=w483) -> ("Ramp Pattern"=w482:dbl[])  [unwired: 7 in, 1 out]
                  n181 = Build Array(w482, "Index 2", "Index 3", "Index 4", "Index 5") -> (w469:T6)
                  n182 = Build Array(w482, "Coeffs 2", "Coeffs 3", "Coeffs 4", "Coeffs 5") -> (w486:T6)
                  n183 = Transpose Matrix(1:w486) -> (0:w479:T6)
                  n184 = Transpose Matrix(1:w469) -> (0:w477:T6)
                  n185 = Array Size(array=w469) -> (size(s)=w470:i32[])
                  n186 = Index Array(array=w470, index=1) -> (element=w476:i32)
                  "# of Phase" <- w476
                  n187 = stacked-sequence {
                    seq-local: [w499 _ _] -> [_ w515 w581]
                    seq-local: [w500 _ _] -> [_ w509 _]
                    seq-local: [_ w508 _] -> [_ _ w578]
                    seq-local: [w498 _ _] -> [_ w507 _]
                    tunnel: w476 -> [_ w518 _]
                    tunnel: w468 -> [w505 _ _]
                    tunnel: w467 -> [w504 w510 _]
                    tunnel: w480 -> [w502 _ _]
                    tunnel: w477 -> [_ w517 _]
                    tunnel: w479 -> [_ w516 _]
                    tunnel: [_ w514 _] -> w478
                    tunnel: w475 -> [_ w512 w579]
                    tunnel: w474 -> [_ w513 w580]
                    tunnel: w473 -> [_ w511 _]
                    tunnel: w472 -> [w501 _ _]
                    tunnel: [_ _ w577] -> w471
                    tunnel: [w499 _ _] -> w466
                    tunnel: w465 -> [_ w506 w575]
                    frame #0 {
                      n188 = local read "interaction matrix file"() -> (w494:path)
                      n189 = local read "Initial haso file"() -> (w495:path)
                      n190 = local read "idxType"() -> (w497:enum16{"Wyant", "ANSI"})
                      n191 = local read "Haso configuration file"() -> (w496:path)
                      n192 = call "zern2command_test.vi"("Haso configuration file"=w496, "idxType"=w497, "Initial haso file"=w495, "error in (no error)"=w501, "interaction matrix file"=w494, "Zern coef in"=w504, "Zern index in"=w505) -> ("error out"=w500:errorcluster, "Zern coef out"=w498:sgl[], "Offset positions"=w503:sgl[])  [unwired: 2 in]
                      n193 = Add(x=w503, y=w502) -> (x+y=w499:dbl[])
                    }
                    frame #1 {
                      n194 = for {
                        N: w518 -> [w521]
                        tunnel: w517 -> [w532] mode=indexing
                        tunnel: w516 -> [w531] mode=indexing
                        tunnel: w515 -> [w530]
                        tunnel: [w529] -> w514 mode=indexing
                        tunnel: w513 -> [w528]
                        tunnel: w512 -> [w527]
                        tunnel: w511 -> [w526]
                        tunnel: w510 -> [w525]
                        tunnel: w509 -> [w524]
                        tunnel: [w523] -> w508
                        tunnel: w507 -> [w520]
                        tunnel: w506 -> [w519]
                        i -> [w522]
                        n195 = stacked-sequence {
                          seq-local: [w542 _] -> [_ w553]
                          seq-local: [w538 _] -> [_ w561]
                          tunnel: w532 -> [w549 _]
                          tunnel: w531 -> [w548 _]
                          tunnel: w530 -> [w546 _]
                          tunnel: [w545 _] -> w529
                          tunnel: w528 -> [_ w563]
                          tunnel: w527 -> [_ w562]
                          tunnel: w526 -> [_ _]
                          tunnel: w522 -> [w544 _]
                          tunnel: w525 -> [w540 _]
                          tunnel: w524 -> [w539 _]
                          tunnel: [_ w560] -> w523
                          tunnel: w522 -> [_ _]
                          tunnel: w521 -> [_ _]
                          tunnel: w520 -> [w537 _]
                          tunnel: w519 -> [_ w557]
                          frame #0 {
                            n196 = Equal To 0?(x=w544) -> (x = 0?=w543:bool)
                            n197 = local read "idxType"() -> (w536:enum16{"Wyant", "ANSI"})
                            n198 = local read "Initial haso file"() -> (w534:path)
                            n199 = local read "interaction matrix file"() -> (w533:path)
                            n200 = local read "Haso configuration file"() -> (w535:path)
                            n201 = call "zern2command_test.vi"("Haso configuration file"=w535, "idxType"=w536, "Initial haso file"=w534, "error in (no error)"=w539, "interaction matrix file"=w533, "Zern coef in"=w548, "Zern index in"=w549) -> ("error out"=w538:errorcluster, "Zern coef out"=w541:sgl[], "Offset positions"=w547:sgl[])  [unwired: 2 in]
                            n202 = case shown="False" w543 {
                              tunnel: [w550 w551] -> w542
                              tunnel: w541 -> [w550 _]
                              tunnel: w540 -> [_ _]
                              tunnel: w537 -> [_ w551]
                              frame False {
                              }
                              frame True {
                              }
                            }
                            n203 = Add(x=w546, y=w547) -> (x+y=w545:dbl[])
                          }
                          frame #1 {
                            n204 = Number To Fractional String(number=w557, precision (6)=0) -> (F-format string=w556:string)  [unwired: 2 in]
                            n205 = Concatenate Strings(w563, w562, "_", w556, "_coeff.txt") -> (w571:string)
                            n206 = String To Path(string=w571) -> (path=w570:path)
                            n207 = Multiply(x=w553, y=1.0) -> (x*y=w552:dbl[])
                            n208 = Open/Create/Replace File(file path (use dialog)=w570, error in=w561, operation (0:open)=3) -> (refnum out=w567:refnum<file>, error out=w568:errorcluster)  [unwired: 3 in, 1 out]
                            n209 = Array To Spreadsheet String(array=w552, 3:"%f") -> (spreadsheet string=w559:string)  [unwired: 1 in]
                            n210 = Set File Position(refnum=w567, from (0:start)=1, error in=w568) -> (refnum out=w565:refnum<file>, error out=w564:errorcluster)  [unwired: 1 in]
                            n211 = Write to Text File(file (use dialog)=w565, text=w559, error in=w564) -> (error out=w560:errorcluster)  [unwired: 1 in, 2 out]
                          }
                        }
                      }
                    }
                    frame #2 {
                      n212 = Number To Fractional String(number=w575, precision (6)=0) -> (F-format string=w574:string)  [unwired: 2 in]
                      n213 = Concatenate Strings(w580, w579, "_", w574, "_IniAbr+offset.txt") -> (w590:string)
                      n214 = String To Path(string=w590) -> (path=w588:path)
                      n215 = Open/Create/Replace File(file path (use dialog)=w588, error in=w578, operation (0:open)=3) -> (refnum out=w585:refnum<file>, error out=w586:errorcluster)  [unwired: 3 in, 1 out]
                      n216 = Array To Spreadsheet String(array=w581, 3:"%f") -> (spreadsheet string=w592:string)  [unwired: 1 in]
                      n217 = Set File Position(refnum=w585, from (0:start)=1, error in=w586) -> (refnum out=w583:refnum<file>, error out=w582:errorcluster)  [unwired: 1 in]
                      n218 = Write to Text File(file (use dialog)=w583, text=w592, error in=w582) -> (error out=w577:errorcluster)  [unwired: 1 in, 2 out]
                    }
                  }
                }
                frame #3 {
                  # "save phase diversity pictures:\npictures per phase*number of phases (Eg: 2*5=10 pictures in this file)"
                  # "readout and delay"
                  # "take phase diversity pictures"
                  n219 = local read "EMCCD trigger port"() -> (w610:tag)
                  n220 = Number To Fractional String(number=w597, precision (6)=0) -> (F-format string=w601:string)  [unwired: 2 in]
                  n221 = Multiply(x=w614, y=1000.0) -> (x*y=w613:dbl)
                  n222 = Concatenate Strings(w595, w594, "_", w601) -> (w596:string)
                  n223 = Add(x=w613, y=50.0) -> (x+y=w606:dbl)
                  n224 = call "applyDM_and_acqTIFF_mCMD.vi"("EMCCD trigger port"=w610, "WavefrontCorrector in"=w609, "Absolute Positions"=w603, "exp and readout time (ms)"=w606, "CMD Num"=w608, "Img Num"=w607, "error in (no error)"=w605, "strPath"=w596, "Clean Spooling"=TRUE, "strPalette"="C:\\Program Files\\Andor SOLIS\\GREY.PAL") -> ("error out"=w604:errorcluster)  [unwired: 4 in, 1 out]
                }
                frame #4 {
                  # "take a picture of groundtruth and offset+ini abbr, and cal imq for each"
                  n225 = stacked-sequence {
                    tunnel: w624 -> [w639 w658]
                    tunnel: w623 -> [w638 w657]
                    tunnel: w622 -> [w637 w656]
                    tunnel: w621 -> [w633 w653]
                    tunnel: w618 -> [_ w645]
                    tunnel: w620 -> [w636 w655]
                    tunnel: w619 -> [w626 w647]
                    tunnel: [w625 _] -> w617
                    tunnel: w616 -> [w635 _]
                    tunnel: [_ w643] -> w615
                    frame #0 {
                      # "calculate imq of groundtruth"
                      # "take a picture of groundtruth"
                      n226 = Number To Fractional String(number=w637, precision (6)=0) -> (F-format string=w640:string)  [unwired: 2 in]
                      n227 = Concatenate Strings(w639, w638, "_grdtrth_", w640) -> (w629:string)
                      n228 = local read "EMCCD trigger port"() -> (w634:tag)
                      n229 = call "applyDM_and_acqTIFF.vi"("EMCCD trigger port"=w634, "WavefrontCorrector in"=w636, "Absolute Positions"=w635, "exp and readout time (ms)"=w633, "Img Num"=1, "strPath"=w629) -> ("error out"=w630:errorcluster)  [unwired: 8 in, 1 out]
                      n230 = Concatenate Strings(w629, ".tif") -> (w628:string)
                      n231 = call "calculate_IQM_MATLAB.vi"("error in (no error)"=w630, "Background Value"=w626, "File Path and Name w/.tif"=w628, "Metrics Type"="Metrics Type") -> ("image quality"=w625:dbl)  [unwired: 6 in, 1 out]
                      "Groundtruth IQM" <- w625
                    }
                    frame #1 {
                      # "take a picture of offset+ini abbr"
                      # "calculate imq of groundtruth"
                      n232 = Number To Fractional String(number=w656, precision (6)=0) -> (F-format string=w659:string)  [unwired: 2 in]
                      n233 = Concatenate Strings(w658, w657, "_abbr_", w659) -> (w649:string)
                      n234 = local read "EMCCD trigger port"() -> (w654:tag)
                      n235 = call "applyDM_and_acqTIFF.vi"("EMCCD trigger port"=w654, "WavefrontCorrector in"=w655, "Absolute Positions"=w645, "exp and readout time (ms)"=w653, "Img Num"=1, "strPath"=w649) -> ("error out"=w650:errorcluster)  [unwired: 8 in, 1 out]
                      n236 = Concatenate Strings(w649, ".tif") -> (w648:string)
                      n237 = local read "Metrics Type"() -> (w646:T4)
                      n238 = call "calculate_IQM_MATLAB.vi"("error in (no error)"=w650, "Background Value"=w647, "File Path and Name w/.tif"=w648, "Metrics Type"=w646) -> ("image quality"=w643:dbl)  [unwired: 6 in, 1 out]
                      "Aberrated IQM" <- w643
                    }
                  }
                }
                frame #5 {
                  # "run matlab correction?"
                  n239 = local read "interaction matrix file"() -> (w664:path)
                  n240 = local read "Initial haso file"() -> (w663:path)
                  n241 = local read "Haso configuration file"() -> (w662:path)
                  n242 = case shown="True" w677 {
                    tunnel: w681 -> [_ w709]
                    tunnel: w682 -> [_ w708]
                    tunnel: w680 -> [_ w707]
                    tunnel: w668 -> [_ w706]
                    tunnel: w679 -> [_ w705]
                    tunnel: w678 -> [_ w704]
                    tunnel: w667 -> [_ w703]
                    tunnel: w676 -> [_ _]
                    tunnel: [0 w702] -> w675
                    tunnel: w674 -> [_ w701]
                    tunnel: [errorcluster {"status"=FALSE, "code"=0, "source"=""} ("Error out 2") w700] -> w673
                    tunnel: w672 -> [_ w699]
                    tunnel: w671 -> [_ w698]
                    tunnel: w670 -> [_ w697]
                    tunnel: w669 -> [_ w694]
                    tunnel: w668 -> [_ w696]
                    tunnel: w667 -> [_ w695]
                    tunnel: w666 -> [_ w693]
                    tunnel: w665 -> [_ w692]
                    tunnel: w664 -> [_ w690]
                    tunnel: w663 -> [_ w689]
                    tunnel: w662 -> [_ w688]
                    tunnel: "Initial Phase Num" -> [_ w687]
                    frame False {
                      n243 = local write "All IQM"(dbl[] []) -> ()
                    }
                    frame True {
                      # "matlab reconstructed Zern"
                      n244 = stacked-sequence {
                        seq-local: [w726 _] -> [_ w852]
                        seq-local: [w728 _] -> [_ w851]
                        tunnel: w709 -> [w727 w871]
                        tunnel: w708 -> [w725 w870]
                        tunnel: w707 -> [w720 w857]
                        tunnel: w706 -> [_ _]
                        tunnel: w704 -> [_ _]
                        tunnel: w705 -> [_ _]
                        tunnel: w703 -> [w724 w869]
                        tunnel: [w723 _] -> w702
                        tunnel: w701 -> [_ w862]
                        tunnel: [_ w849] -> w700
                        tunnel: w699 -> [w715 w855]
                        tunnel: w698 -> [_ _]
                        tunnel: w697 -> [w722 _]
                        tunnel: w696 -> [w719 w863]
                        tunnel: w695 -> [w718 _]
                        tunnel: w687 -> [w721 _]
                        tunnel: w694 -> [w717 _]
                        tunnel: w693 -> [w716 _]
                        tunnel: w692 -> [_ _]
                        tunnel: [w714 _] -> w691
                        tunnel: w690 -> [w713 w853]
                        tunnel: w689 -> [w712 w848]
                        tunnel: w688 -> [w711 w847]
                        tunnel: [w710 _] -> w686
                        frame #0 {
                          n245 = while {
                            tunnel: [w751] -> w728
                            tunnel: w727 -> [w750]
                            tunnel: [w749] -> w726
                            tunnel: w725 -> [w748]
                            tunnel: w724 -> [w747]
                            tunnel: [w746] -> w723
                            tunnel: w722 -> [w745]
                            shift-right: [w737] -> _
                            shift-left: w721 -> [w744]
                            tunnel: w720 -> [w743]
                            tunnel: w719 -> [w742]
                            tunnel: w718 -> [w741]
                            tunnel: w717 -> [w740]
                            tunnel: w716 -> [w735]
                            tunnel: w715 -> [w734]
                            tunnel: [w733] -> w714 mode=indexing
                            tunnel: w713 -> [w732]
                            tunnel: w712 -> [w731]
                            tunnel: w711 -> [w730]
                            tunnel: [w729] -> w710 mode=indexing
                            stop <- w738 stop-if-true
                            n246 = stacked-sequence {
                              seq-local: [w765 _ _] -> [_ w808 _]
                              seq-local: [w764 _ _] -> [_ w816 _]
                              tunnel: [w764 _ _] -> w751
                              tunnel: w750 -> [w782 w818 _]
                              tunnel: [w765 _ _] -> w749
                              tunnel: w748 -> [w762 w817 _]
                              tunnel: w747 -> [w777 _ _]
                              tunnel: [w756 _ _] -> w746
                              tunnel: w745 -> [w766 w795 _]
                              tunnel: w744 -> [w753 w813 w834]
                              tunnel: w743 -> [_ w815 _]
                              tunnel: w742 -> [_ w803 _]
                              tunnel: w741 -> [_ w814 _]
                              tunnel: w740 -> [_ w793 _]
                              tunnel: [_ w796 _] -> w739
                              tunnel: [_ _ w833] -> w737
                              tunnel: [_ _ w832] -> w736
                              tunnel: w735 -> [_ _ _]
                              tunnel: w734 -> [_ w806 _]
                              tunnel: [_ w791 _] -> w733
                              tunnel: w732 -> [_ w811 _]
                              tunnel: w731 -> [_ w810 _]
                              tunnel: w730 -> [_ w809 _]
                              tunnel: [w753 _ _] -> w729
                              frame #0 {
                                w759 = "_"
                                n247 = local read "idxType"() -> (w755:enum16{"Wyant", "ANSI"})
                                n248 = Number To Fractional String(number=w777, precision (6)=0) -> (F-format string=w758:string)  [unwired: 2 in]
                                n249 = Concatenate Strings(w762, "_", w758) -> (w767:string)
                                n250 = String To Path(string=w782) -> (path=w783:path)
                                n251 = Number To Fractional String(number=w753, precision (6)=0) -> (F-format string=w761:string)  [unwired: 2 in]
                                n252 = Concatenate Strings(w782, w762, w759, w761, "ImgCorr", w759, w758) -> (w781:string)
                                n253 = case shown="\"ANSI\"" w755 {
                                tunnel: [2 3] -> w754
                                frame "Wyant", Default {
                                }
                                frame "ANSI" {
                                }
                                }
                                n254 = String To Path(string=w781) -> (path=w780:path)
                                n255 = call "recon_zern_fileIO_MATLAB_v2.vi"("Number of Phase"=w753, "Number for average"="Num for average", "Crop Size of image"="Crop Size of image", "Background Value"=w766, "Zernike Order"="Zernike Index Limit", "Use GPU"="Use GPU", "Iteration Number"="Max Iteration Num", "idxType"=w755, "File Name"=w767, "Gamma Value"="Gamma Value", "Path In"=w783, "Show Input"="Show Input", "Path Out"=w780, "Show Recon"="Show Recon") -> ("Zern coef out"=w752:sgl[], "Time cost (s)"=→"Recon Time (s)":dbl, "RMSE Value"=w756:dbl, "error out"=w764:errorcluster)  [unwired: 10 in]
                                "RMSE Value" <- w756
                                "Zern coeffs recon" <- w752
                                n256 = case shown="True" "Apply Defocus" {
                                tunnel: w752 -> [w786 w790]
                                tunnel: [w786 w788] -> w765
                                tunnel: w754 -> [_ w787]
                                frame False {
                                }
                                frame True {
                                n257 = Replace Array Subset(array=w790, new element=0.0, index=w787) -> (w788:sgl[])
                                }
                                }
                                "Recon Img Num" <- w753
                              }
                              frame #1 {
                                w826 = 1
                                # "get correction command\ntake a picture"
                                n258 = Number To Fractional String(number=w813, precision (6)=0) -> (F-format string=w819:string)  [unwired: 2 in]
                                n259 = Array Size(array=w808) -> (size(s)=w807:i32)
                                n260 = Number To Fractional String(number=w814, precision (6)=0) -> (F-format string=w822:string)  [unwired: 2 in]
                                n261 = call-poly <vilib>:"Ramp Pattern.vi"("start"=w826, "end"=w807, "delta"=w826) -> ("Ramp Pattern"=w825:dbl[])  [unwired: 6 in, 2 out]
                                n262 = Concatenate Strings(w818, w817, "_", w819, "ImgCorr_", w822) -> (w797:string)
                                n263 = local read "idxType"() -> (w812:enum16{"Wyant", "ANSI"})
                                n264 = call "zern2command_test.vi"("Haso configuration file"=w809, "idxType"=w812, "Initial haso file"=w810, "error in (no error)"=w816, "interaction matrix file"=w811, "Zern coef in"=w808, "Zern index in"=w825) -> ("error out"=w798:errorcluster, "Offset positions"=w824:sgl[])  [unwired: 2 in, 1 out]
                                n265 = Subtract(x=w815, y=w824) -> (x-y=w804:dbl[])
                                n266 = call "applyDM_and_acqTIFF.vi"("WavefrontCorrector in"=w806, "Absolute Positions"=w804, "exp and readout time (ms)"=w803, "Img Num"=1, "error in (no error)"=w798, "strPath"=w797) -> ("error out"=w794:errorcluster)  [unwired: 8 in, 1 out]
                                n267 = Concatenate Strings(w797, ".tif") -> (w802:string)
                                n268 = local read "Metrics Type"() -> (w801:T4)
                                n269 = call "calculate_IQM_MATLAB.vi"("error in (no error)"=w794, "Background Value"=w795, "File Path and Name w/.tif"=w802, "Metrics Type"=w801) -> ("image quality"=w791:dbl)  [unwired: 6 in, 1 out]
                                "Corrected IQM" <- w791
                                n270 = case shown="False" "Auto Stop" {
                                tunnel: [FALSE w830] -> w796
                                tunnel: w791 -> [_ w829]
                                tunnel: w793 -> [_ w828]
                                frame False {
                                }
                                frame True {
                                n271 = Greater?(x=w829, y=w828) -> (0:w830:bool)
                                }
                                }
                              }
                              frame #2 {
                                n272 = case shown="\"Progressive Feedback\"" "Feedback Type" {
                                tunnel: w834 -> [w837 w839 w841]
                                tunnel: [w837 w838 w842] -> w833
                                tunnel: [TRUE w840 w844] -> w832
                                tunnel: "Final Phase Num" -> [_ w838 w843]
                                frame "Single Correction", Default {
                                }
                                frame "One Step Feedback" {
                                n273 = Greater Or Equal?(x=w839, y=w838) -> (x >= y?=w840:bool)
                                }
                                frame "Progressive Feedback" {
                                n274 = Increment(x=w841) -> (x+1=w842:u32)
                                n275 = Greater Or Equal?(x=w841, y=w843) -> (x >= y?=w844:bool)
                                }
                                }
                              }
                            }
                            n276 = Or(x=w739, y=w736) -> (x .or. y?=w738:bool)
                          }
                        }
                        frame #1 {
                          w861 = 1
                          # "set andor kinetics and spooling, \nstart acquire and wait for the external trigger"
                          n277 = Array Size(array=w852) -> (size(s)=w858:i32)
                          n278 = call-poly <vilib>:"Ramp Pattern.vi"("start"=w861, "end"=w858, "delta"=w861) -> ("Ramp Pattern"=w860:dbl[])  [unwired: 6 in, 2 out]
                          n279 = local read "idxType"() -> (w854:enum16{"Wyant", "ANSI"})
                          n280 = call "zern2command_test.vi"("Haso configuration file"=w847, "idxType"=w854, "Initial haso file"=w848, "error in (no error)"=w851, "interaction matrix file"=w853, "Zern coef in"=w852, "Zern index in"=w860) -> ("error out"=w850:errorcluster, "Offset positions"=w859:sgl[])  [unwired: 2 in, 1 out]
                          n281 = Subtract(x=w857, y=w859) -> (x-y=w856:dbl[])
                          n282 = Build Array(w862, w857, w856) -> (w846:T6)
                          n283 = Number To Fractional String(number=w869, precision (6)=0) -> (F-format string=w872:string)  [unwired: 2 in]
                          n284 = Transpose Matrix(1:w846) -> (0:w845:T6)
                          n285 = local read "EMCCD trigger port"() -> (w864:tag)
                          n286 = Concatenate Strings(w871, w870, "_grdtrth_abrr_Corr_", w872) -> (w868:string)
                          n287 = call "applyDM_and_acqTIFF_mCMD.vi"("EMCCD trigger port"=w864, "WavefrontCorrector in"=w855, "Absolute Positions"=w845, "exp and readout time (ms)"=w863, "CMD Num"=3, "Img Num"=1, "error in (no error)"=w850, "strPath"=w868) -> ("error out"=w849:errorcluster)  [unwired: 6 in, 1 out]
                        }
                      }
                      "All IQM" <- w691
                      "Img Num Used" <- w686
                    }
                  }
                }
                frame #6 {
                  # "save image quality values"
                  n288 = local read "File Base Name"() -> (w881:string)
                  n289 = local read "Output path"() -> (w882:path)
                  n290 = Number To Fractional String(number=w899, precision (6)=0) -> (F-format string=w888:string)  [unwired: 2 in]
                  n291 = Concatenate Strings(w888, ".txt") -> (w879:string)
                  n292 = local read "Img Num Used"() -> (w898:dbl[])
                  n293 = local read "All IQM"() -> (w897:dbl[])
                  n294 = local read "Groundtruth IQM"() -> (w896:dbl)
                  n295 = local read "Aberrated IQM"() -> (w895:dbl)
                  n296 = Concatenate Strings(w881, "_IQM_InitialAber_", w879) -> (w887:string)
                  n297 = Build Array(w898, w897) -> (w883:T6)
                  n298 = Concatenate Strings(w881, "_IQM_Corrected_", w879) -> (w878:string)
                  n299 = Build Array(w896, w895) -> (w891:dbl[])
                  n300 = Build Path(base path=w882, name or relative path=w887) -> (appended path=w892:path)
                  n301 = Array To Spreadsheet String(array=w891, 3:"%f") -> (spreadsheet string=w893:string)  [unwired: 1 in]
                  n302 = Build Path(base path=w882, name or relative path=w878) -> (appended path=w884:path)
                  n303 = Array To Spreadsheet String(array=w883, 3:"%f") -> (spreadsheet string=w885:string)  [unwired: 1 in]
                  n304 = Write to Text File(file (use dialog)=w892, text=w893) -> (refnum out=w875:refnum<file>, error out=w874:errorcluster)  [unwired: 2 in, 1 out]
                  n305 = Write to Text File(file (use dialog)=w884, text=w885) -> (refnum out=w877:refnum<file>, error out=w876:errorcluster)  [unwired: 2 in, 1 out]
                  n306 = Close File(refnum=w875, error in=w874) -> ()  [unwired: 2 out]
                  n307 = Close File(refnum=w877, error in=w876) -> ()  [unwired: 2 out]
                }
              }
            }
          }
          frame #2 {
            # "shut down shutter of 488nm laser"
            n308 = invoke class="MG17Motor" method="SC_Disable"(reference=w904, "lChanID"=w903) -> (reference out=w902:refnum<k7>, "lChanID"=w901:i32)  [unwired: 2 in, 2 out]
          }
          frame #3 {
            # "save the RMS of (calculated zer-real zer)"
            n309 = Concatenate Strings(w907, w906, "_RMSE.txt") -> (w912:string)
            n310 = String To Path(string=w912) -> (path=w911:path)
            n311 = Number To Fractional String(number=w908) -> (F-format string=w909:string[])  [unwired: 3 in]
            n312 = Write to Text File(file (use dialog)=w911, text=w909) -> (error out=w905:errorcluster)  [unwired: 2 in, 2 out]
          }
        }
        n313 = Merge Errors(w382, w381, w376) -> (w375:errorcluster)
        "Error out" <- w375
        n314 = Unbundle(w375) -> ("status"=w371:bool)  [unwired: 2 out]
        n315 = case shown="False" w371 {
          tunnel: [w398 w399] -> w374
          tunnel: w371 -> [w397 w399]
          frame False {
            n316 = Not(x=w397) -> (.not. x?=w398:bool)
          }
          frame True {
          }
        }
        n317 = Or(x=w374, y="?") -> (x .or. y?=w372:bool)
      }
    }
    frame #4 {
      n318 = case shown="True" "Turn off EMCCD when finished?" {
        frame False {
        }
        frame True {
          n319 = flat-sequence {
            frame #0 {
              n320 = call <userlib>:"CoolerOFF.vi"() -> ()  [unwired: 2 in, 2 out]
            }
            frame #1 {
              # "shut down EMCCD"
              n321 = call <userlib>:"ShutDown.vi"() -> ()  [unwired: 2 in, 2 out]
            }
          }
        }
      }
    }
    frame #5 {
      # "if not \"stop control\", the shutter can be control when the program is not running"
      # "shut down casao"
      n322 = call <userlib>:"LVClass_WavefrontCorrector dtor.vi"("WavefrontCorrector in"=w918, "error in (no error)"=w916) -> ("error out"=w915:errorcluster)  [unwired: 12 in, 1 out]
      n323 = call <userlib>:"LVClass_WavefrontCorrectorSet dtor.vi"("WavefrontCorrectorSet in"=w917, "error in (no error)"=w915) -> ()  [unwired: 12 in, 2 out]
      n324 = case shown="True" FALSE {
        tunnel: w919 -> [_ w920]
        frame False {
        }
        frame True {
          n325 = invoke class="MG17Motor" method="StopCtrl"(reference=w920) -> ()  [unwired: 2 in, 3 out]
        }
      }
    }
  }
  n326 = local read "Metrics Type"() -> (w1:T4)
  n327 = case shown="\"sharpness - image domain\"" w1 {
    tunnel: [" \" \", Default." " \"max intensity\"." " \"mean intensity\"." " \"RMS contrast\"." " \"sharpness - image domain\"." " \"sharpness - spectral domain 1: 0~r0\"." " \"sharpness - spectral domain 2: 0.1*r0~0.5*r0\"." " \"norm DCT  - spectral domain 3: 0~r0\"."] -> _
    frame " ", Default {
    }
    frame "max intensity" {
    }
    frame "mean intensity" {
    }
    frame "RMS contrast" {
    }
    frame "sharpness - image domain" {
    }
    frame "sharpness - spectral domain 1: 0~r0" {
    }
    frame "sharpness - spectral domain 2: 0.1*r0~0.5*r0" {
    }
    frame "norm DCT  - spectral domain 3: 0~r0" {
    }
  }
